vi "VP_NanoPositioner_FPGA_MultiScan.vi"() -> ()   [LabVIEW 2015]
uses:
  FPGA states.ctl
  FPGA Commands.ctl
  RT VIs/Scan type.ctl
  <vilib>/Platform/TimedLoop/XDataNode/timing_clust.ctl
  <vilib>/Platform/TimedLoop/XDataNode/nitl_modes.ctl
  <vilib>/Platform/TimedLoop/XDataNode/wakeup.ctl
  Control X Up Down Ramp.ctl
  Detector_Trigger_Control.ctl
  Control Y Up Down Ramp.ctl
  <vilib>/rvi/Emulation/niFpgaGetClockAttributes.vi
  <vilib>/rvi/Emulation/niFpgaSctlEmulationGetInTimedLoop.vi
  <vilib>/rvi/Emulation/niFpgaEmulationReportErrorSimple.vi
  <vilib>/rvi/Emulation/niFpgaProcessEmulError.vi
  <vilib>/rvi/Emulation/niFpgaCriticalErrorInLSC.vi
  <vilib>/rvi/interface/RandomDataEmulation/niFpgaRandomDataHandleErrors.vi
  <vilib>/rvi/eio/common/nirviEmuTemplateMethod_errors.vi
  <vilib>/rvi/DataTransferAndStorage/Container/XNode/niFpgaContainer.xnode
  <vilib>/rvi/interface/RandomDataEmulation/nirviRandomDataFpgaReadWriteTemplate.vi
  <vilib>/eio/EIONode/EIONode.xnode
  <vilib>/rvi/Analysis/measure/butterworth/XNode/niFpgaButterworthFilter.xnode
  <vilib>/Platform/TimedLoop/XDataNode/XDataNode.xnode
  <vilib>/Platform/TimedLoop/XDataNode/XDNodeRunTimeDep.lvlib
panel:
  in  "Scan type":T1
  out "Interferometer Loop Error":errorcluster
  out "Fly scan completed":bool
  out "Y scan done":bool=TRUE
  out "X scan done":bool=TRUE
  out "Wait error":errorcluster
  out "Shutdown error":errorcluster
  out "FPGA error monitor":errorcluster
  out "Run Loop error":errorcluster
  in  "Wait timer (ms)":u16=50 caption="Count(mSec)"
  in  "New FPGA command":bool
  in  "FPGA command":T2
  out "FPGA state":T3
  out "End Run Error":errorcluster
  out "Measured Data Trigger Time Period (Ticks)":u32
  in  "Data Trigger Time Period (uSec)":u32 caption="Detector Trigger Time Period (uSec)"
  out "Trigger for Data":fxp<+/-,58,25>
  out "Fly Scan Running":bool
  in  "Fly Scan":bool
  out "If True End Y Down Ramp":bool
  in  "Y Ramp Drop Size (nm)":fxp<+/-,16,16>
  out "Ramp Mid Range":bool
  out "If True End Up Ramp":bool
  out "Start or middle":bool=TRUE
  in  "Y Start Marker (nm)":fxp<+/-,58,25> format="%#_55g"
  out "Y Ramp Slope":fxp<+,48,16>
  in  "Y Ramp End (nm)":fxp<+/-,16,16>
  in  "Y Ramp Start (nm)":fxp<+/-,16,16>
  in  "Y Ramp Period (usec)":fxp<+,32,32>
  in  "X Ramp Period (usec)":fxp<+,32,32>
  in  "X Ramp End (nm)":fxp<+/-,16,16>
  in  "X Ramp Start (nm)":fxp<+/-,16,16>
  out "If True End X Down Ramp":bool
  out "X Ramp Mid Range":bool
  out "If True End X Up Ramp":bool
  out "Y Ramp Drop":bool
  out "Next Do Down Ramp":bool
  out "Continue Run":bool
  in  "X Start Marker (nm)":fxp<+/-,58,25>
  out "X Ramp Slope":fxp<+,48,16> format="%.37g"
  in  "DT Reset":bool
  in  "DT Duty Cycle (periods)":fxp<+,32,0>=0.5 caption="DT duty cycle (periods)"
  in  "DT Reference DC Offset (V)":fxp<+/-,16,16>
  in  "DT Reference Amplitude (V)":fxp<+/-,40,17>
  in  "DT Phase Offset (periods)":fxp<+,32,0>
  in  "DT Frequency (periods/tick)":fxp<+,32,0>=0.0002500000409781933
  in  "Trigger Wave Generator":T4(ring)
  out "If True End Trigger Low":bool
  in  "Trigger Low Level (V)":fxp<+/-,20,5>=-5.0
  in  "Trigger High Level (V)":fxp<+/-,20,5>=5.0
  out "If True End Trigger High":bool
  out "Trigger Mid High":bool
  in  "Trigger Low Period (usec)":fxp<+/-,64,45>
  in  "Trigger High Period (usec)":fxp<+/-,64,45>
  out "Measured Z Reference Time Period (Ticks)":u32
  in  "Z Reference Time Period (uSec)":u32
  in  "Z White Noise Amplitude":u16=32767
  in  "Z White Noise Seed":u32=4
  in  "Z Phase Offset (periods)":fxp<+,32,0>
  in  "Z Frequency (periods/tick)":fxp<+,32,0>=0.0002500000409781933
  in  "Z Reference DC Offset (nm)":fxp<+/-,16,16>
  in  "Z Reference Amplitude (nm)":fxp<+/-,40,17>
  in  "Z Reference Reset":bool
  in  "Z Reference Wave Selection":T5(ring)
  in  "Y White Noise Amplitude":u16=32767
  in  "Y White Noise Seed":u32=4
  out "Measured Y Reference Time Period (Ticks)":u32
  in  "Y Reference Time Period (uSec)":u32
  in  "Y Reference Reset":bool
  in  "Y Reference Wave Selection":T6(ring)
  in  "Detector Trigger Lower Limit (V)":fxp<+/-,20,5>=-5.0
  out "Detector Trigger In Range?":bool
  in  "Detector Trigger Upper Limit (V)":fxp<+/-,20,5>=5.0
  out "Detector Trigger (V)":fxp<+/-,20,5> format="%.29g"
  out "Measured Detector Trigger Time Period (Ticks)":u32
  in  "Detector Trigger Time Period (uSec)":u32
  out "Measured Trigger Gen Time Period (Ticks)":u32
  in  "Trigger Generation Time Period (uSec)":u32
  in  "Reference Signal Source":T7(ring)
  in  "Z-Stage Scaling Direction":fxp<+/-,3,3>=-1.0
  in  "Y-Stage Scaling Direction":fxp<+/-,3,3>=-1.0
  in  "Y Phase Offset (periods)":fxp<+,32,0>
  in  "Y Frequency (periods/tick)":fxp<+,32,0>=0.0002500000409781933
  in  "Optics and or Sample Stage":T8(ring)
  out "Z Stage External Reference (nm)":fxp<+/-,58,25>
  in  "Mod 3 AI2 V to nm Scaling":fxp<+,47,18>
  out "Mod 8 Input AI2 (V)":fxp<+/-,24,5>
  out "Y Stage External Reference (nm)":fxp<+/-,58,25>
  in  "Mod 3 AI1 V to nm Scaling":fxp<+,47,18>
  out "Mod 8 Input AI1 (V)":fxp<+/-,24,5>
  in  "Sample Z Stage Resolution (nm)":fxp<+,33,3>=0.001000046730041504
  in  "Sample Y Stage Resolution (nm)":fxp<+,33,3>=0.001000046730041504
  in  "Sample X Stage Resolution (nm)":fxp<+,33,3>=0.001000046730041504
  out "Sample Z Stage Displacement (nm)":fxp<+/-,58,25>
  out "Sample Z Stage Displacement raw (nm)":fxp<+/-,64,35> format="%.62g"
  out "Sample Y Stage Displacement (nm)":fxp<+/-,58,25>
  out "Sample Y Stage Displacement raw (nm)":fxp<+/-,64,35> format="%.41g"
  out "Sample X Stage Displacement raw (nm)":fxp<+/-,64,35> format="%.62g"
  out "Sample X Stage Displacement (nm)":fxp<+/-,58,25>
  in  "Reset Sample Z":bool
  out "32 bit Count Sample  Z":i32
  in  "Reset Sample Y":bool
  out "32 bit Count Sample  Y":i32
  in  "Reset Sample X":bool
  out "32 bit Count Sample X":i32
  out "Mod6/DIO3":bool
  out "Mod6/DIO2":bool
  out "Mod5/DIO3":bool
  out "Mod5/DIO2":bool
  out "Mod4/DIO3":bool
  out "Mod4/DIO2":bool
  out "Measured Analog Input Time Period (Ticks)":u32
  in  "Analog Input Time Period (uSec)":u32
  out "X Stage External Reference (nm)":fxp<+/-,58,25>
  in  "Mod 3 AI0 V to nm Scaling":fxp<+,47,18>
  out "Mod 3 Input AI0 (V)":fxp<+/-,24,5>
  in  "X-Stage Scaling Direction":fxp<+/-,3,3>=-1.0
  in  "Z-Stage nm to V Scaling":fxp<+/-,32,12>
  in  "Y-Stage nm to V Scaling":fxp<+/-,32,12>
  in  "X-Stage nm to V Scaling":fxp<+/-,32,12>
  out "Kxx Output, Kxx*ex (V)":fxp<+/-,58,25>
  out "Kyy Output, Kyy*ey (V)":fxp<+/-,58,25>
  out "Kzz Output, Kzz*ez (V)":fxp<+/-,58,25>
  in  "sos gain SF Controller xx1":fxp<+/-,42,9>
  in  "-a01(2) xx1":fxp<+/-,64,9>[](array[numeric])=[0.0, 0.0, 0.0, 0.0, 0.0, 0.0, 0.0, 0.0, 0.0, 0.0, 0.0, 0.0, 0.0, 0.0, 0.0, 0.0, 0.0, 0.0, 0.0, 0.0]
  in  "-a02(2) xx1":fxp<+/-,64,9>[](array[numeric])=[0.0, 0.0, 0.0, 0.0, 0.0, 0.0, 0.0, 0.0, 0.0, 0.0, 0.0, 0.0, 0.0, 0.0, 0.0, 0.0, 0.0, 0.0, 0.0, 0.0]
  in  "b01(2) xx1":fxp<+/-,64,9>[](array[numeric])=[0.0, 0.0, 0.0, 0.0, 0.0, 0.0, 0.0, 0.0, 0.0, 0.0, 0.0, 0.0, 0.0, 0.0, 0.0, 0.0, 0.0, 0.0, 0.0, 0.0]
  in  "b02(2) xx1":fxp<+/-,64,9>[](array[numeric])=[0.0, 0.0, 0.0, 0.0, 0.0, 0.0, 0.0, 0.0, 0.0, 0.0, 0.0, 0.0, 0.0, 0.0, 0.0, 0.0, 0.0, 0.0, 0.0, 0.0]
  in  "sos gain SF Controller yy1":fxp<+/-,42,9>
  in  "-a01(2) yy1":fxp<+/-,64,9>[](array[numeric])=[0.0, 0.0, 0.0, 0.0, 0.0, 0.0, 0.0, 0.0, 0.0, 0.0, 0.0, 0.0, 0.0, 0.0, 0.0, 0.0, 0.0, 0.0, 0.0, 0.0]
  in  "-a02(2) yy1":fxp<+/-,64,9>[](array[numeric])=[0.0, 0.0, 0.0, 0.0, 0.0, 0.0, 0.0, 0.0, 0.0, 0.0, 0.0, 0.0, 0.0, 0.0, 0.0, 0.0, 0.0, 0.0, 0.0, 0.0]
  in  "b01(2) yy1":fxp<+/-,64,9>[](array[numeric])=[0.0, 0.0, 0.0, 0.0, 0.0, 0.0, 0.0, 0.0, 0.0, 0.0, 0.0, 0.0, 0.0, 0.0, 0.0, 0.0, 0.0, 0.0, 0.0, 0.0]
  in  "b02(2) yy1":fxp<+/-,64,9>[](array[numeric])=[0.0, 0.0, 0.0, 0.0, 0.0, 0.0, 0.0, 0.0, 0.0, 0.0, 0.0, 0.0, 0.0, 0.0, 0.0, 0.0, 0.0, 0.0, 0.0, 0.0]
  in  "sos gain SF Controller zz1":fxp<+/-,42,9>
  in  "-a01(2) zz1":fxp<+/-,64,9>[](array[numeric])=[0.0, 0.0, 0.0, 0.0, 0.0, 0.0, 0.0, 0.0, 0.0, 0.0, 0.0, 0.0, 0.0, 0.0, 0.0, 0.0, 0.0, 0.0, 0.0, 0.0]
  in  "-a02(2) zz1":fxp<+/-,64,9>[](array[numeric])=[0.0, 0.0, 0.0, 0.0, 0.0, 0.0, 0.0, 0.0, 0.0, 0.0, 0.0, 0.0, 0.0, 0.0, 0.0, 0.0, 0.0, 0.0, 0.0, 0.0]
  in  "b01(2) zz1":fxp<+/-,64,9>[](array[numeric])=[0.0, 0.0, 0.0, 0.0, 0.0, 0.0, 0.0, 0.0, 0.0, 0.0, 0.0, 0.0, 0.0, 0.0, 0.0, 0.0, 0.0, 0.0, 0.0, 0.0]
  in  "b02(2) zz1":fxp<+/-,64,9>[](array[numeric])=[0.0, 0.0, 0.0, 0.0, 0.0, 0.0, 0.0, 0.0, 0.0, 0.0, 0.0, 0.0, 0.0, 0.0, 0.0, 0.0, 0.0, 0.0, 0.0, 0.0]
  in  "Scaling mV to V":fxp<+,33,10>=0.0009765625
  in  "System Loop Type":enum16{"Open Loop", "Closed Loop"}(ring)
  in  "Timeout FPGA FIFO1":i32=40000000
  out "FIFO Timed Out":bool
  out "Number of Data Strings":i32
  in  "Y Reference DC Offset (nm)":fxp<+/-,16,16>
  in  "X Reference DC Offset (nm)":fxp<+/-,16,16>
  in  "Y Reference Amplitude (nm)":fxp<+/-,40,17>
  out "Z Stage Reference (nm)":fxp<+/-,58,25> format="%.41g"
  out "Y Stage Reference (nm)":fxp<+/-,58,25> format="%.41g"
  out "Optics Z Stage Displacement (nm)":fxp<+/-,58,25>
  out "Optics Z Stage Displacement raw (nm)":fxp<+/-,64,35>
  in  "Optics Z Stage Resolution (nm)":fxp<+,33,3>=0.001000046730041504
  in  "Reset Optics Z":bool
  out "32 bit Count Optics  Z":i32
  out "Mod6/DIO1":bool
  out "Mod6/DIO0":bool
  out "Optics Y Stage Displacement (nm)":fxp<+/-,58,25>
  out "Optics Y Stage Displacement raw (nm)":fxp<+/-,64,35>
  in  "Optics Y Stage Resolution (nm)":fxp<+,33,3>=0.001000046730041504
  in  "Reset Optics Y":bool
  out "32 bit Count Optics  Y":i32
  out "Mod5/DIO1":bool
  out "Mod5/DIO0":bool
  out "Z-Stage Input In Range?":bool
  out "Y-Stage Input In Range?":bool
  in  "Controller Output Lower Limit":fxp<+/-,20,5>=-5.0
  out "X-Stage Input In Range?":bool
  in  "Controller Output Upper Limit":fxp<+/-,20,5>=5.0
  in  "X White Noise Amplitude":u16=32767
  in  "X White Noise Seed":u32=4
  in  "X Reference Reset":bool
  in  "X Reference Wave Selection":T9(ring)
  out "Measured Counter Time Period (Ticks)":u32
  out "Measured Datalog Time Period (Ticks)":u32
  out "Measured Plant Output Time Period (Ticks)":u32
  out "Measured Controller Output Time Period (Ticks)":u32
  out "Measured Controller Time Period (Ticks)":u32
  out "Measured X Reference Time Period (Ticks)":u32
  out "Optics X Stage Displacement raw (nm)":fxp<+/-,64,35>
  in  "Optics X Stage Resolution (nm)":fxp<+,33,3>=0.001000046730041504 format="%#_31g"
  in  "Plant Output Time Period (uSec)":u32
  out "Optics X Stage Displacement (nm)":fxp<+/-,58,25>
  in  "Reset Optics X":bool
  out "32 bit Count Optics X":i32
  out "Mod4/DIO1":bool
  out "Mod4/DIO0":bool
  out "Start Run Error":errorcluster
  out "stop case":bool
  in  "Controller Output Time Period (uSec)":u32
  in  "Datalog Cases":T10(ring)
  out "PI Z-Stage Input (V)":fxp<+/-,20,5> format="%.29g"
  out "PI Y-Stage Input (V)":fxp<+/-,20,5> format="%.29g"
  out "PI X-Stage Input (V)":fxp<+/-,20,5> format="%.29g"
  in  "Controller Time Period (uSec)":u32
  in  "Datalog Time Period (uSec)":u32
  in  "X Reference Time Period (uSec)":u32
  in  "X Reference Amplitude (nm)":fxp<+/-,40,17>
  out "X Stage Reference (nm)":fxp<+/-,58,25> format="%.41g"
  out "FIFO Timed Out?":bool
  in  "X Phase Offset (periods)":fxp<+,32,0>
  in  "X Frequency (periods/tick)":fxp<+,32,0>=0.0002500000409781933
types:
  T1 = typedef "Scan type.ctl" = enum16{"Fly", "Step"}
  T2 = typedef "FPGA Commands.ctl" = enum16{"Start Scan", "Shutdown"}
  T3 = typedef "FPGA states.ctl" = enum16{"Wait", "Start Run", "Run", "End Run", "Shutdown"}
  T4 = enum16{"Custom Square Wave ", "Square Wave 1", "Square Wave 2"}
  T5 = enum16{"Constant", "Sine Wave", "Sawtooth Wave", "Square Wave", "Filtered White Noise"}
  T6 = enum16{"Constant", "Sine Wave", "Custom Ramp Wave", "Filtered White Noise"}
  T7 = enum16{"FPGA Generated Reference", "External Reference"}
  T8 = enum16{"Optics Stage Only", "Optics and Sample Stage"}
  T9 = enum16{"Constant", "Sine Wave", "Custom Up Down Ramp", "Filtered White Noise"}
  T10 = enum16{"Data Log 1", "Data Log 2", "Data Log 3", "Data Log 4", "Data Log 5", "Data Log 6", "Data Log 7", "Data Log 8", "Data Log 9", "Data Log 10", "Data Log 11", "Data Log 12", "Data Log 13", "Data Log 14", "Data Log 15", "Data Log 16"}
  T11 = typedef "Control Y Up Down Ramp.ctl" = enum16{"Y Up Ramp", "Y Down Ramp"}
  T12 = typedef "Detector_Trigger_Control.ctl" = enum16{"Trigger High", "Trigger Low"}
  T13 = typedef "Control X Up Down Ramp.ctl" = enum16{"X Up Ramp", "X Down Ramp"}
  T14 = typedef "XDNodeRunTimeDep.lvlib/timing_clust.ctl" = cluster{"Expected End [f-1]":u64, "Actual End [f-1]":u64, "Finished Late? [f-1]":bool, "Expected End [i-1]":u64, "Actual End [i-1]":u64, "Finished Late? [i-1]":bool, "Expected Start [i]":u64, "Actual Start [i]":u64, "Expected Start [f]":u64, "Actual Start [f]":u64, "Source Name":string, "Structure Name":string, "Period":i64, "Deadline":i64, "Offset":i64, "Start":i64, "Priority":i32, "Timeout":i32, "Mode":T15, "Wakeup Reason":T16, "Error":errorcluster, "Source Type":string, "Secondary Source Type":string, "Global End Time":u64, "Global Start Time":u64, "Frame Duration":u64, "Iteration Duration":u64, "Assigned CPU":i32, "I/O Scan Engine Mode":u32}
  T15 = typedef "XDNodeRunTimeDep.lvlib/nitl_modes.ctl" = enum32{"No Change", "Process missed periods, maintain original phase", "Discard missed periods, maintain original phase", "Process missed periods, ignore original phase", "Discard missed periods, ignore original phase"}
  T16 = typedef "XDNodeRunTimeDep.lvlib/wakeup.ctl" = enum32{"Normal", "Aborted", "Asynchronous wakeup", "Timing source error", "Timed loop error", "Timeout"}
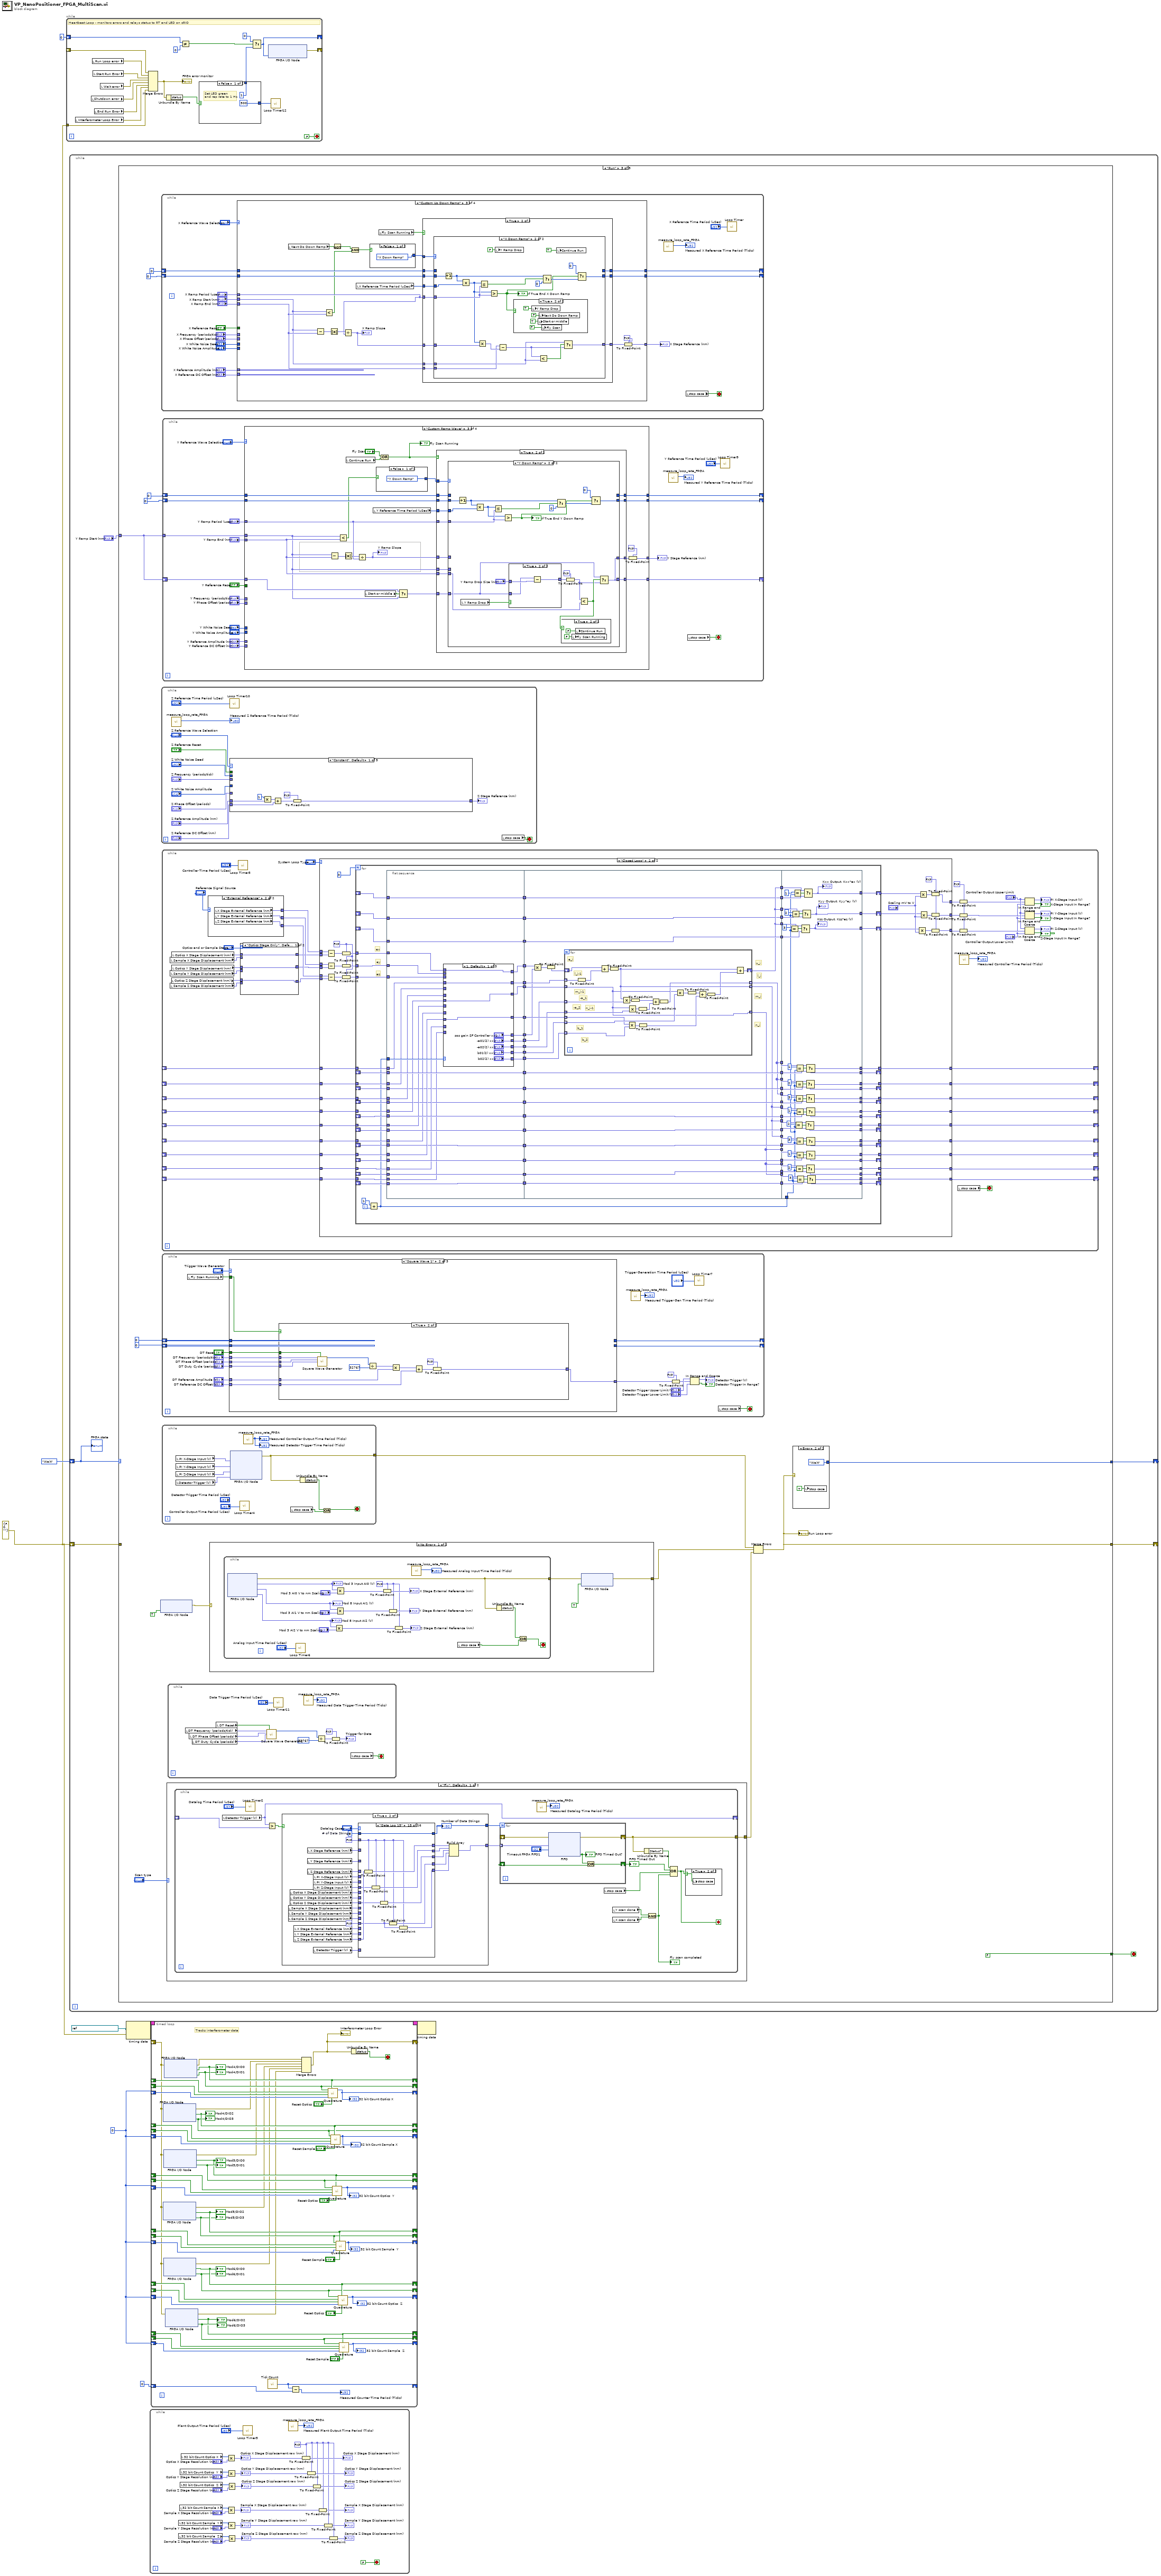
[diagram p0: block diagram]
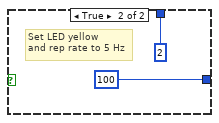
[diagram p2: hidden frame]
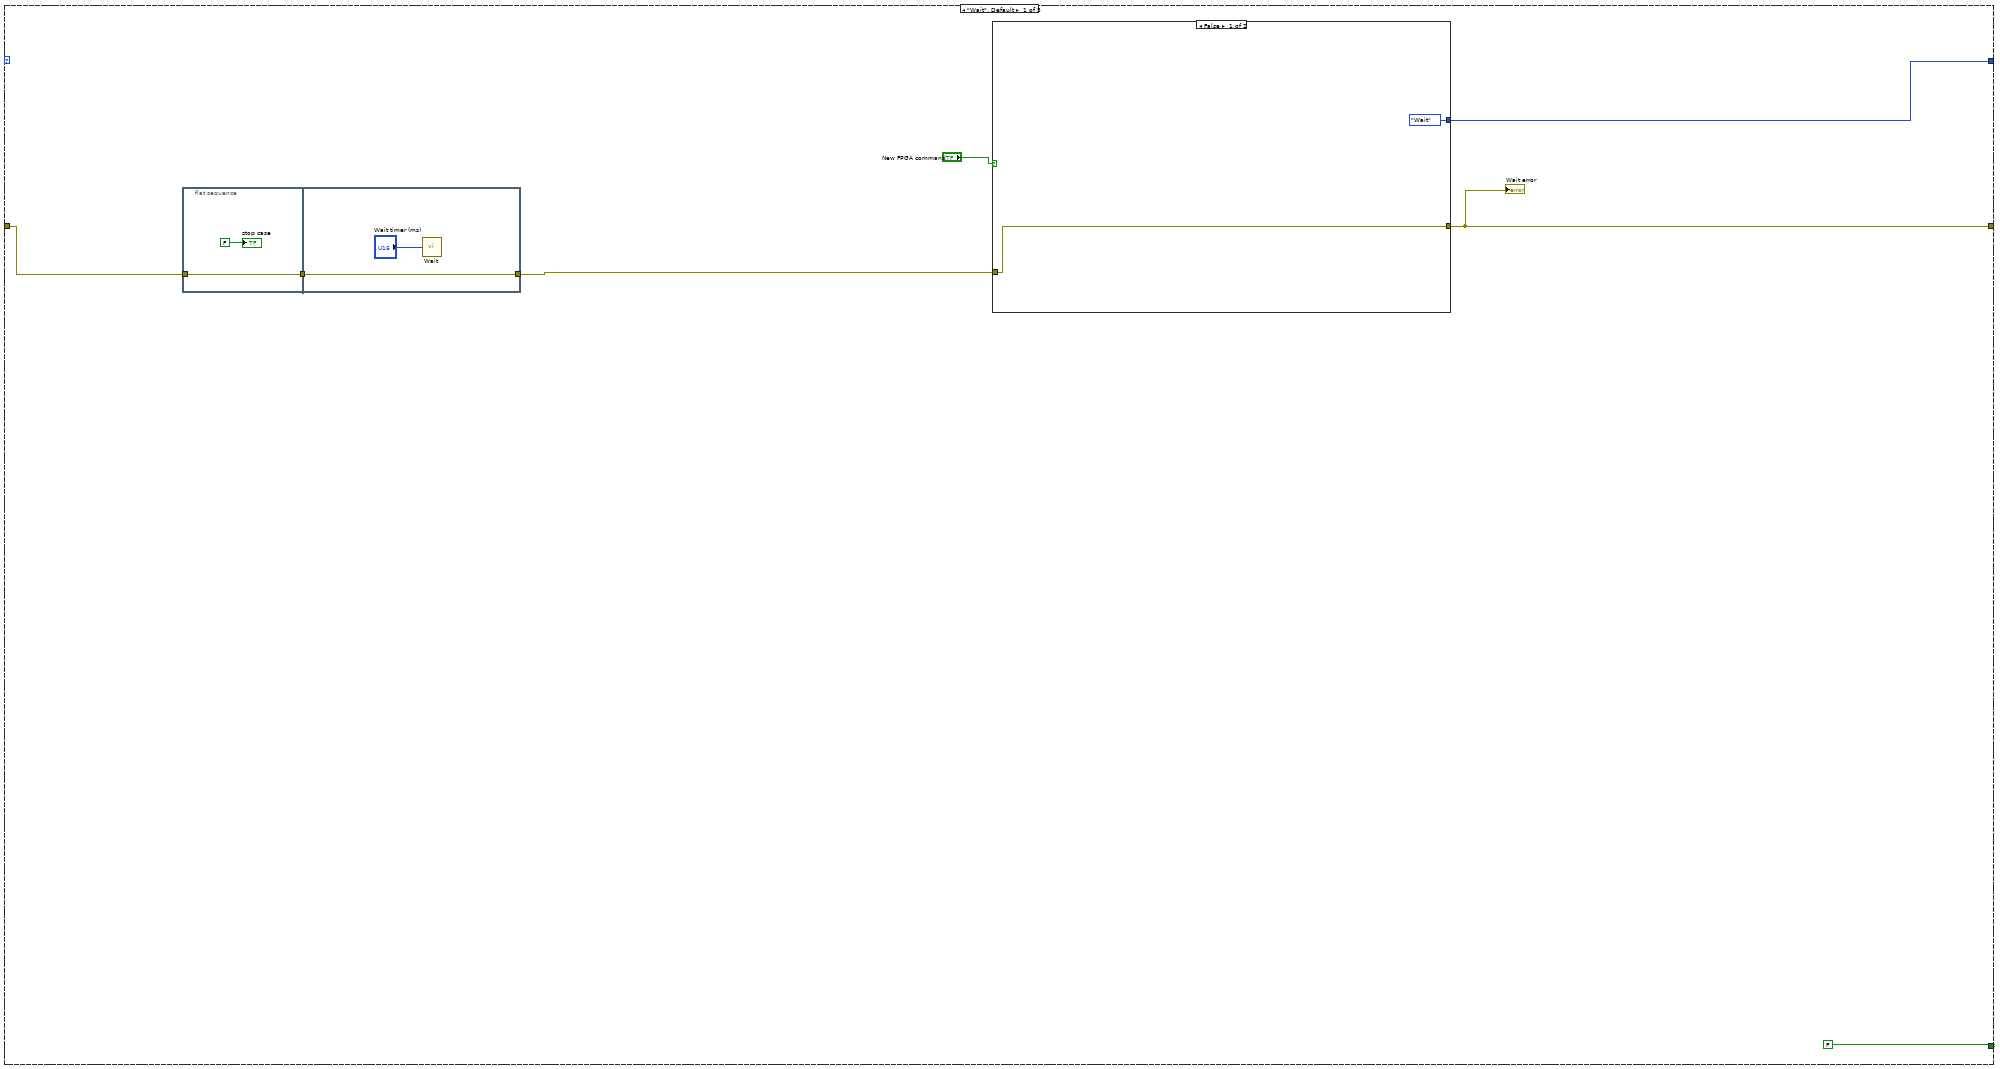
[diagram p3: hidden frame]
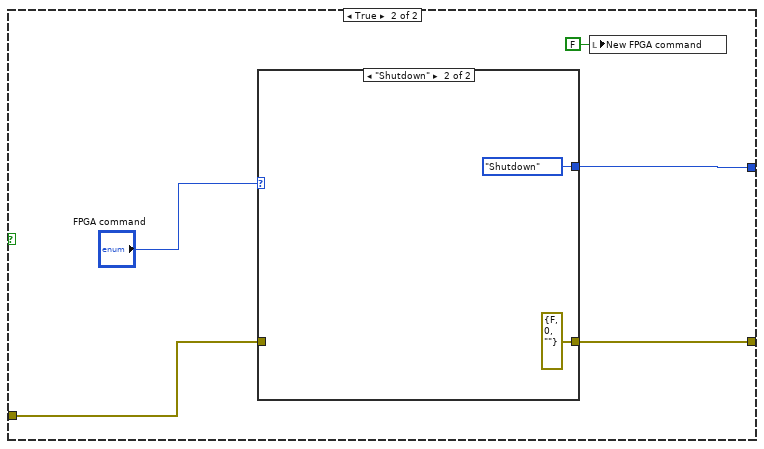
[diagram p4: hidden frame]
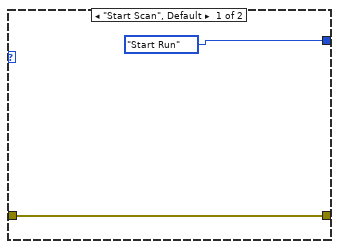
[diagram p5: hidden frame]
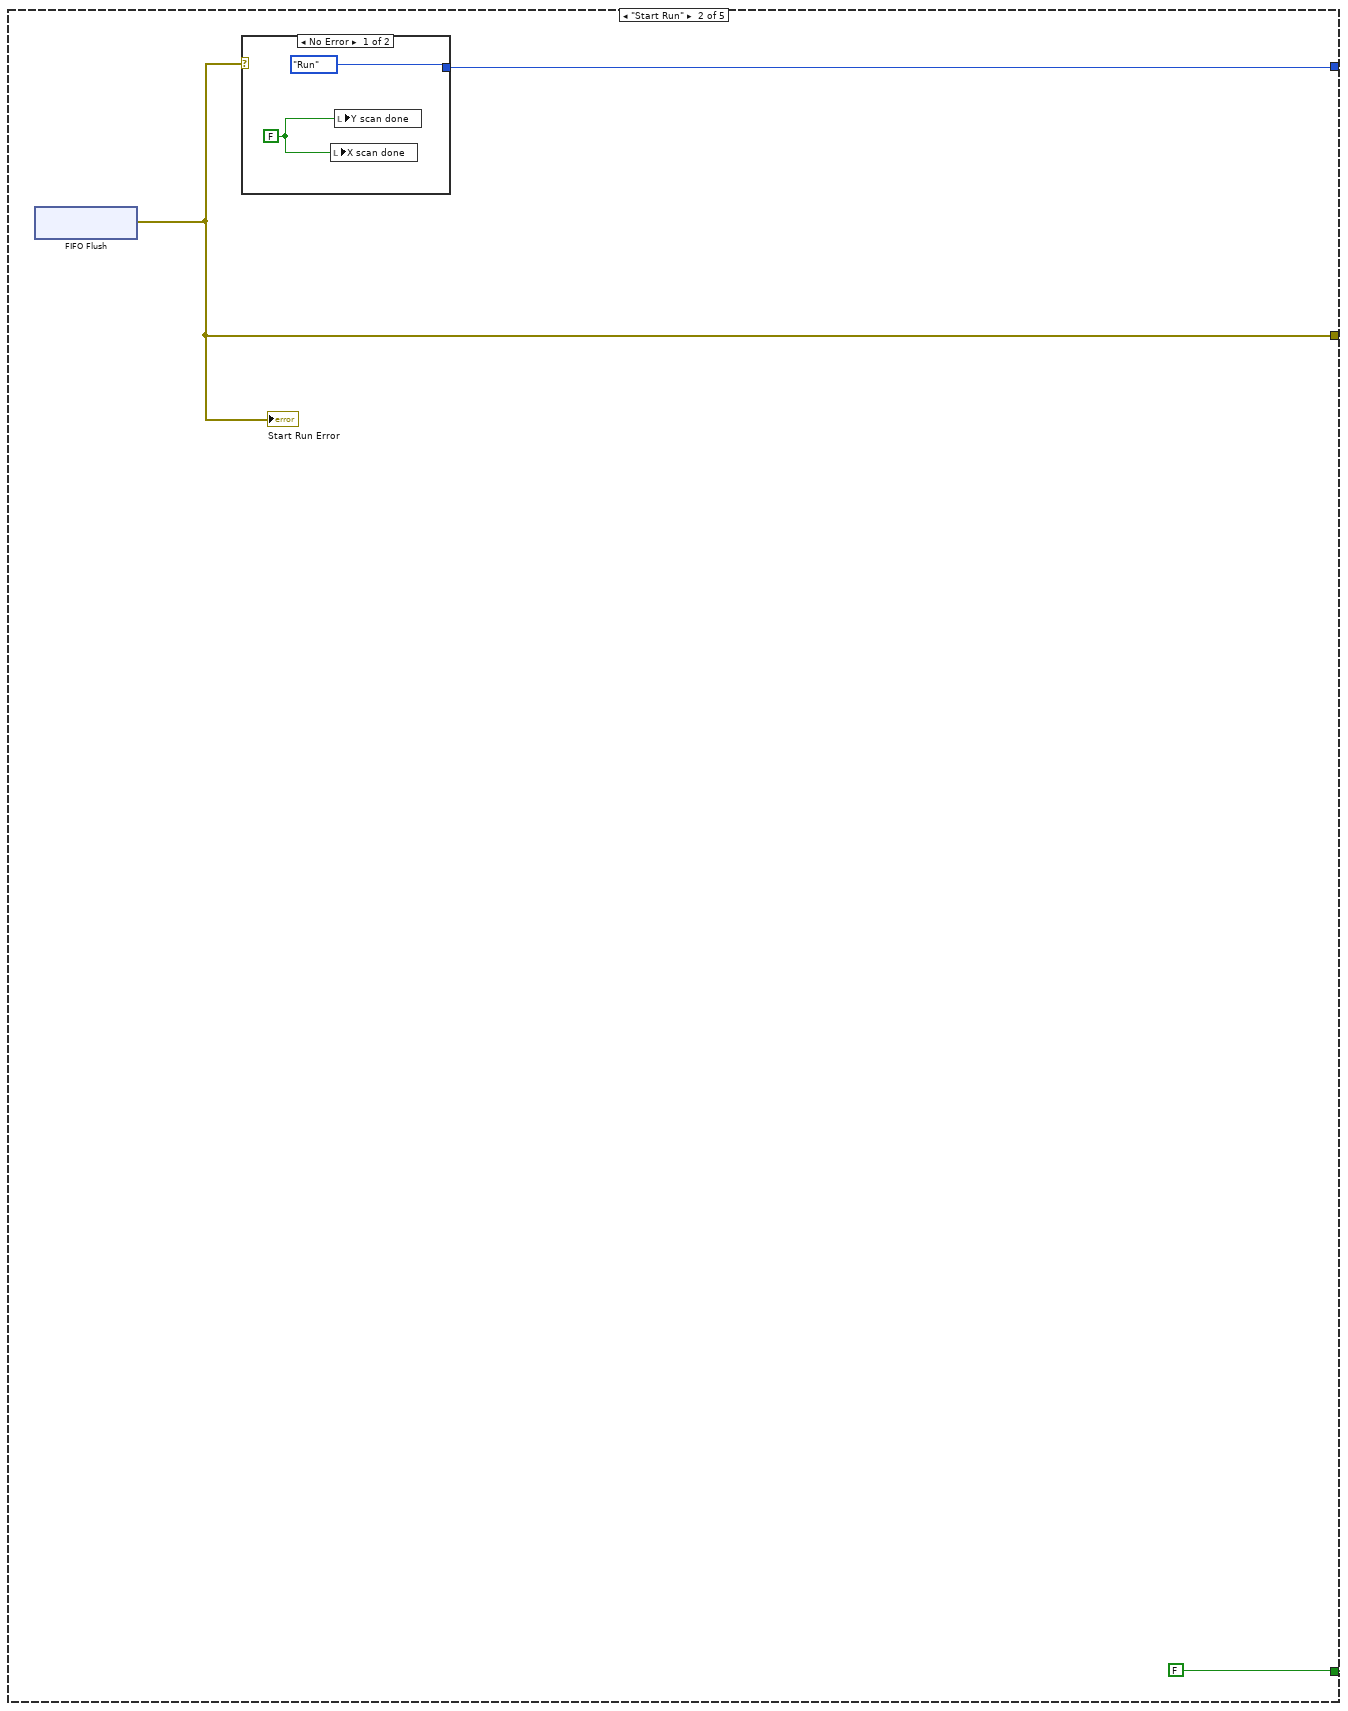
[diagram p6: hidden frame]
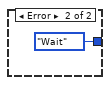
[diagram p7: hidden frame]
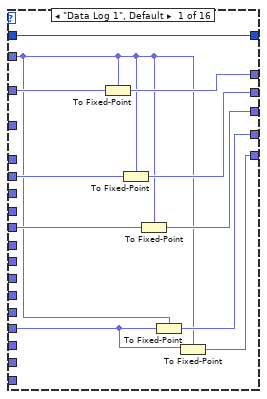
[diagram p10: hidden frame]
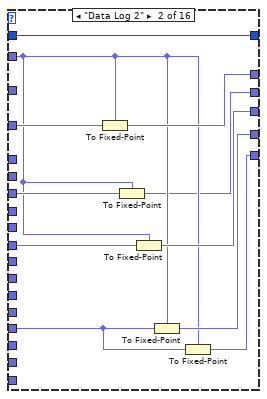
[diagram p11: hidden frame]
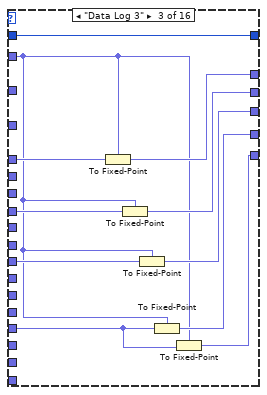
[diagram p12: hidden frame]
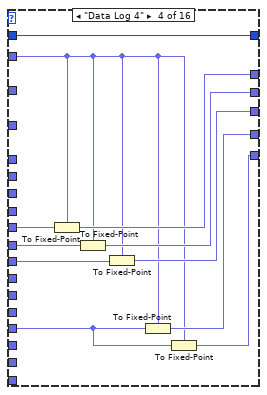
[diagram p13: hidden frame]
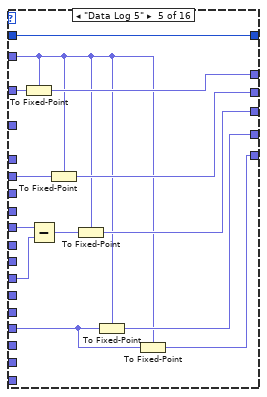
[diagram p14: hidden frame]
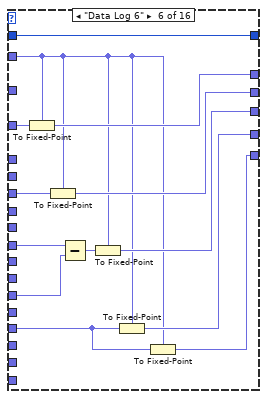
[diagram p15: hidden frame]
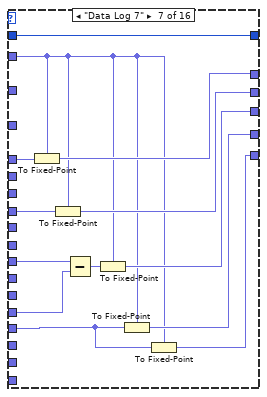
[diagram p16: hidden frame]
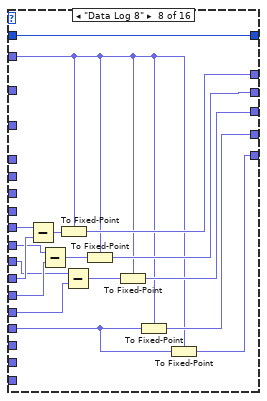
[diagram p17: hidden frame]
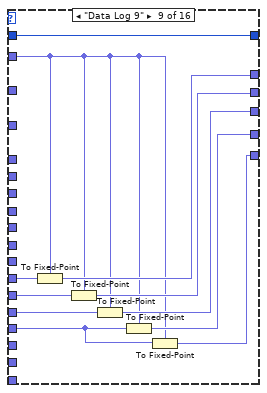
[diagram p18: hidden frame]
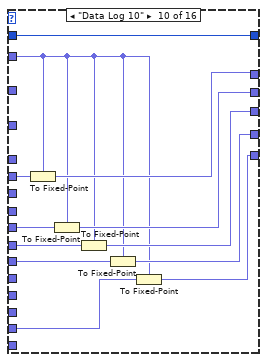
[diagram p19: hidden frame]
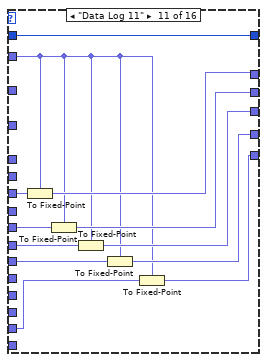
[diagram p20: hidden frame]
diagram:
  w4 = 0 ("Tick Count(Ticks)")
  w1 = errorcluster {"status"=FALSE, "code"=0, "source"=""} ("error IO")
  n1 = while {
    tunnel: w1 -> [w22]
    shift-right: [w20] -> _
    shift-left: _ -> [w19]
    shift-right: [w17] -> _
    shift-left: u8 0 ("USER FPGA LED") -> [w15]
    stop <- FALSE stop-if-true
    # "Heartbeat Loop - monitors errors and relays status to RT and LED on cRIO"
    n2 = local read "Interferometer Loop Error"() -> (w9:errorcluster)
    n3 = local read "Shutdown error"() -> (w24:errorcluster)
    n4 = local read "Run Loop error"() -> (w27:errorcluster)
    n5 = local read "Start Run Error"() -> (w26:errorcluster)
    n6 = local read "End Run Error"() -> (w23:errorcluster)
    n7 = local read "Wait error"() -> (w25:errorcluster)
    n8 = Merge Errors(w19, w27, w26, w25, w24, w23, w9, w22) -> (w21:errorcluster)
    "FPGA error monitor" <- w21
    n9 = Unbundle By Name(w21) -> ("status"=w10:bool)
    n10 = Not Equal?(x=w15, y=u8 0) -> (x != y?=w13:bool)
    n11 = case shown="False" w10 {
      tunnel: [u16 500 ("Count(mSec)") u16 100 ("Count(mSec)")] -> w18
      tunnel: [u8 1 ("USER FPGA LED") u8 2 ("USER FPGA LED")] -> w11
      frame False {
        # "Set LED green \nand rep rate to 1 Hz"
      }
      frame True {
        # "Set LED yellow \nand rep rate to 5 Hz"
      }
    }
    n12 = Select(t=u8 0, s=w13, f=w11) -> (s? t:f=w17:u8)
    n13 = xnode "FPGA I/O Node"("USER FPGA LED"=w17) -> ("error out"=w20:errorcluster)  [unwired: 2 in, 1 out]
    n14 = call "Loop Timer12"("Count(mSec)"=w18) -> ()  [unwired: 1 out]
  }
  n15 = while {
    shift-right: [w35] -> _
    shift-left: FPGA_states."Wait" -> [w37]
    shift-right: [w32] -> _
    shift-left: w1 -> [w34]
    stop <- w36 stop-if-true
    n16 = case shown="\"Run\"" w37 {
      tunnel: [w43 w60 w71 w1303 w1307] -> w32
      tunnel: [FALSE FALSE FALSE FALSE TRUE] -> w36
      tunnel: [w38 w61 w72 FPGA_states."Wait" FPGA_states."Shutdown"] -> w35
      tunnel: w34 -> [w40 _ _ w1303 w1308]
      tunnel: "Y Ramp Start (nm)" -> [_ _ w69 _ _]
      frame "Wait", Default {
        n17 = flat-sequence {
          tunnel: w40 -> [w45]
          tunnel: [w45] -> w41
          tunnel: [w47] -> w39
          tunnel: w41 -> [w47]
          frame #0 {
            "stop case" <- FALSE ("stop case")
          }
          frame #1 {
            n18 = call "Wait"("Count(mSec)"="Wait timer (ms)") -> ()  [unwired: 1 out]
          }
        }
        n19 = case shown="False" "New FPGA command" {
          tunnel: [FPGA_states."Wait" w55] -> w38
          tunnel: w39 -> [w50 w54]
          tunnel: [w50 w53] -> w43
          frame False {
          }
          frame True {
            n20 = case shown="\"Shutdown\"" "FPGA command" {
              tunnel: [FPGA_states."Start Run" FPGA_states."Shutdown"] -> w55
              tunnel: w54 -> [w56 _]
              tunnel: [w56 errorcluster {"status"=FALSE, "code"=0, "source"=""} ("error IO")] -> w53
              frame "Start Scan", Default {
              }
              frame "Shutdown" {
              }
            }
            n21 = local write "New FPGA command"(FALSE ("New FPGA command")) -> ()
          }
        }
        "Wait error" <- w43
      }
      frame "Start Run" {
        n22 = xnode ("FIFO Flush")() -> ("error out"=w60:errorcluster)  [unwired: 2 in, 1 out]
        "Start Run Error" <- w60
        n23 = case shown="No Error" w60 {
          tunnel: [FPGA_states."Run" FPGA_states."Wait"] -> w61
          frame No Error {
            w63 = FALSE
            n24 = local write "X scan done"(w63) -> ()
            n25 = local write "Y scan done"(w63) -> ()
          }
          frame Error {
          }
        }
      }
      frame "Run" {
        n26 = xnode "FPGA I/O Node"("Mod3/Start"=TRUE ("I/O Item")) -> ("error out"=w67:errorcluster)  [unwired: 2 in, 1 out]
        n27 = while {
          shift-right: [w1165] -> _
          shift-left: u32 0 ("f") -> [w1163]
          shift-right: [w1164] -> _
          shift-left: u32 0 -> [w1162]
          stop <- w1174 stop-if-true
          n28 = case shown="\"Custom Up Down Ramp\"" "X Reference Wave Selection" {
            tunnel: "X Frequency (periods/tick)" -> [_ w1196 _ _]
            tunnel: "X Phase Offset (periods)" -> [_ w1195 _ _]
            tunnel: "X Reference Reset" -> [_ w1193 _ w1292]
            tunnel: "X White Noise Seed" -> [_ _ _ w1294]
            tunnel: "X White Noise Amplitude" -> [_ _ _ w1291]
            tunnel: "X Reference Amplitude (nm)" -> [w1181 w1188 _ w1282]
            tunnel: "X Reference DC Offset (nm)" -> [w1180 w1187 _ w1283]
            tunnel: [w1179 w1186 w1200 w1285] -> w1167
            tunnel: [_ _ w1213 _] -> w1165
            tunnel: [_ _ w1212 _] -> w1164
            tunnel: w1163 -> [_ _ w1211 _]
            tunnel: w1162 -> [_ _ w1210 _]
            tunnel: "X Ramp Period (usec)" -> [_ _ w1209 _]
            tunnel: "X Ramp Start (nm)" -> [_ _ w1198 _]
            tunnel: "X Ramp End (nm)" -> [_ _ w1199 _]
            frame "Constant", Default {
              n29 = Multiply(x=i16 1 ("y"), y=w1181) -> (x*y=w1184:fxp<+/-,56,33>)
              n30 = Add(x=w1184, y=w1180) -> (x+y=w1183:fxp<+/-,56,33>)
              n31 = To Fixed-Point(fixed-point type=fxp<+/-,58,25> 0.0, number=w1183) -> (fixed-point=w1179:fxp<+/-,58,25>)
            }
            frame "Sine Wave" {
              n32 = call "Sine Wave Generator"("frequency (periods/tick)"=w1196, "reset"=w1193, "phase offset (periods)"=w1195) -> ("sine out"=w1194:i16)  [unwired: 12 in]
              n33 = Divide(x=w1194, y=i16 32767) -> (x/y=w1189:fxp<+/-,41,18>)
              n34 = Multiply(x=w1189, y=w1188) -> (x*y=w1191:fxp<+/-,64,35>)
              n35 = Add(x=w1191, y=w1187) -> (x+y=w1190:fxp<+/-,64,36>)
              n36 = To Fixed-Point(fixed-point type=fxp<+/-,58,25> 0.0, number=w1190) -> (fixed-point=w1186:fxp<+/-,58,25>)
            }
            frame "Custom Up Down Ramp" {
              n37 = local read "Next Do Down Ramp"() -> (w1205:bool)
              n38 = Subtract(x=w1198, y=w1199) -> (x-y=w1215:fxp<+/-,17,17>)
              n39 = Less?(x=w1198, y=w1199) -> (x < y?=w1204:bool)
              n40 = Absolute Value(x=w1215) -> (abs(x)=w1214:fxp<+,16,16>)
              n41 = Not(x=w1205) -> (.not. x?=w1206:bool)
              n42 = Divide(x=w1214, y=w1209) -> (x/y=w1216:fxp<+,48,16>)
              "X Ramp Slope" <- w1216
              n43 = Compound Arithmetic op=AND(w1206, w1204) -> (w1207:bool)
              n44 = local read "X Reference Time Period (uSec)"() -> (w1208:u32)
              n45 = case shown="False" w1207 {
                tunnel: [Control_X_Up_Down_Ramp."X Down Ramp" Control_X_Up_Down_Ramp."X Up Ramp"] -> w1203
                frame False {
                }
                frame True {
                }
              }
              n46 = local read "Fly Scan Running"() -> (w1202:bool)
              n47 = case shown="True" w1202 {
                tunnel: w1203 -> [_ w1233]
                tunnel: w1208 -> [_ w1232]
                tunnel: ["X Start Marker (nm)" w1231] -> w1201
                tunnel: w1209 -> [_ w1230]
                tunnel: w1216 -> [_ w1229]
                tunnel: w1198 -> [_ w1228]
                tunnel: w1199 -> [_ w1227]
                tunnel: [_ w1226] -> w1213
                tunnel: [_ w1225] -> w1212
                tunnel: w1211 -> [_ w1224]
                tunnel: w1210 -> [_ w1223]
                frame False {
                  n48 = local write "Next Do Down Ramp"(FALSE ("Restart Up Ramp")) -> ()
                  n49 = local write "Y Ramp Drop"(FALSE ("Y Toggle 1")) -> ()
                  "X scan done" <- TRUE
                }
                frame True {
                  n50 = case shown="\"X Down Ramp\"" w1233 {
                    tunnel: [w1252 _] -> w1226
                    tunnel: w1224 -> [w1251 _]
                    tunnel: w1232 -> [w1248 w1273]
                    tunnel: w1230 -> [w1247 w1269]
                    tunnel: w1228 -> [w1238 w1260]
                    tunnel: w1227 -> [w1236 w1261]
                    tunnel: [_ w1276] -> w1225
                    tunnel: w1223 -> [_ w1275]
                    tunnel: w1229 -> [w1243 w1267]
                    tunnel: [w1240 w1263] -> w1231
                    frame "X Up Ramp", Default {
                      n51 = Increment(x=w1251) -> (x+1=w1249:u32)
                      n52 = Multiply(x=w1249, y=w1248) -> (x*y=w1244:u32)
                      n53 = Multiply(x=w1244, y=w1243) -> (x*y=w1242:fxp<+,64,48>)
                      n54 = Less Or Equal?(x=w1244, y=w1247) -> (x <= y?=w1246:bool)
                      "X Ramp Mid Range" <- w1246
                      n55 = Add(x=w1242, y=w1238) -> (x+y=w1241:fxp<+/-,64,50>)
                      n56 = Greater?(x=w1244, y=w1247) -> (0:w1237:bool)
                      "If True End X Up Ramp" <- w1237
                      n57 = local write "Y Ramp Drop"(FALSE ("Y Ramp Drop")) -> ()
                      n58 = case shown="True" w1237 {
                        frame False {
                        }
                        frame True {
                          n59 = local write "Start or middle"(TRUE ("Start or middle")) -> ()
                          n60 = local write "Fly Scan"(FALSE ("Fly Scan Start")) -> ()
                          "Y Ramp Drop" <- TRUE ("Boolean")
                          "Next Do Down Ramp" <- TRUE
                        }
                      }
                      n61 = Greater?(x=w1241, y=w1236) -> (0:w1239:bool)
                      n62 = Select(t=w1249, s=w1246, f=u32 0) -> (s? t:f=w1250:u32)
                      n63 = Select(t=w1236, s=w1239, f=w1241) -> (s? t:f=w1240:fxp<+/-,64,50>)
                      n64 = Select(t=u32 0, s=w1237, f=w1250) -> (s? t:f=w1252:u32)
                      "Continue Run" <- TRUE ("Fly Scan Running")
                    }
                    frame "X Down Ramp" {
                      n65 = Increment(x=w1275) -> (x+1=w1274:u32)
                      n66 = Multiply(x=w1274, y=w1273) -> (x*y=w1268:u32)
                      n67 = Multiply(x=w1268, y=w1267) -> (x*y=w1266:fxp<+,64,48>)
                      n68 = Less Or Equal?(x=w1268, y=w1269) -> (x <= y?=w1272:bool)
                      n69 = Greater?(x=w1268, y=w1269) -> (0:w1262:bool)
                      "If True End X Down Ramp" <- w1262
                      n70 = local write "Y Ramp Drop"(FALSE ("Y Ramp Drop")) -> ()
                      n71 = Subtract(x=w1261, y=w1266) -> (x-y=w1264:fxp<+/-,64,50>)
                      n72 = case shown="True" w1262 {
                        frame False {
                        }
                        frame True {
                          n73 = local write "Y Ramp Drop"(TRUE ("Start Scan")) -> ()
                          n74 = local write "Start or middle"(TRUE ("Start or middle")) -> ()
                          n75 = local write "Next Do Down Ramp"(FALSE ("Next Do Down Ramp")) -> ()
                          n76 = local write "Fly Scan"(FALSE ("Fly Scan Start")) -> ()
                        }
                      }
                      n77 = Less?(x=w1264, y=w1260) -> (x < y?=w1265:bool)
                      n78 = Select(t=w1274, s=w1272, f=u32 0) -> (s? t:f=w1270:u32)
                      n79 = local write "Continue Run"(TRUE ("Fly Scan Running")) -> ()
                      n80 = Select(t=w1260, s=w1265, f=w1264) -> (s? t:f=w1263:fxp<+/-,64,50>)
                      n81 = Select(t=u32 0, s=w1262, f=w1270) -> (s? t:f=w1276:u32)
                    }
                  }
                }
              }
              n82 = To Fixed-Point(fixed-point type=fxp<+/-,58,25> 0.0, number=w1201) -> (fixed-point=w1200:fxp<+/-,58,25>)
            }
            frame "Filtered White Noise" {
              n83 = call "White Noise Generator"("seed"=w1294, "reset"=w1292, "amplitude"=w1291) -> ("white noise out"=w1293:i16)  [unwired: 12 in]
              n84 = xnode "Butterworth Filter"("input data"=w1293, "reset"=w1292) -> ("output data"=w1289:i16)  [unwired: 1 in]
              n85 = Divide(x=w1289, y=i16 32767) -> (x/y=w1284:fxp<+/-,41,18>)
              n86 = Multiply(x=w1284, y=w1282) -> (x*y=w1287:fxp<+/-,64,35>)
              n87 = Add(x=w1287, y=w1283) -> (x+y=w1286:fxp<+/-,64,36>)
              n88 = To Fixed-Point(fixed-point type=fxp<+/-,58,25> 0.0, number=w1286) -> (fixed-point=w1285:fxp<+/-,58,25>)
            }
          }
          "X Stage Reference (nm)" <- w1167
          n89 = call "measure_loop_rate_FPGA.vi"() -> ("Loop Rate (Ticks)"=→"Measured X Reference Time Period (Ticks)":u32)  [unwired: 11 in]
          n90 = local read "stop case"() -> (w1174:bool)
          n91 = call "Loop Timer"("Count(uSec)"="X Reference Time Period (uSec)") -> ()  [unwired: 1 out]
        }
        n92 = while {
          stop <- w364 stop-if-true
          n93 = call "measure_loop_rate_FPGA.vi"() -> ("Loop Rate (Ticks)"=→"Measured Z Reference Time Period (Ticks)":u32)  [unwired: 11 in]
          n94 = call "Loop Timer10"("Count(uSec)"="Z Reference Time Period (uSec)") -> ()  [unwired: 1 out]
          n95 = case shown="\"Constant\", Default" "Z Reference Wave Selection" {
            tunnel: "Z Reference Reset" -> [_ w394 w401 w417 w450]
            tunnel: "Z Frequency (periods/tick)" -> [_ w393 w400 w416 _]
            tunnel: "Z Phase Offset (periods)" -> [_ w392 w399 w415 _]
            tunnel: "Z White Noise Seed" -> [_ _ _ _ w452]
            tunnel: "Z White Noise Amplitude" -> [_ _ _ _ w451]
            tunnel: "Z Reference DC Offset (nm)" -> [w376 w385 w396 w407 w441]
            tunnel: "Z Reference Amplitude (nm)" -> [w377 w386 w395 w409 w442]
            tunnel: [w378 w383 w397 w412 w440] -> w365
            frame "Constant", Default {
              n96 = Multiply(x=i16 1 ("y"), y=w377) -> (x*y=w381:fxp<+/-,56,33>)
              n97 = Add(x=w381, y=w376) -> (x+y=w380:fxp<+/-,56,33>)
              n98 = To Fixed-Point(fixed-point type=fxp<+/-,58,25> 0.0, number=w380) -> (fixed-point=w378:fxp<+/-,58,25>)
            }
            frame "Sine Wave" {
              n99 = call "Sine Wave Generator2"("frequency (periods/tick)"=w393, "reset"=w394, "phase offset (periods)"=w392) -> ("sine out"=w387:i16)  [unwired: 12 in]
              n100 = Divide(x=w387, y=i16 32767) -> (x/y=w390:fxp<+/-,41,18>)
              n101 = Multiply(x=w390, y=w386) -> (x*y=w389:fxp<+/-,64,35>)
              n102 = Add(x=w389, y=w385) -> (x+y=w388:fxp<+/-,64,36>)
              n103 = To Fixed-Point(fixed-point type=fxp<+/-,58,25> 0.0, number=w388) -> (fixed-point=w383:fxp<+/-,58,25>)
            }
            frame "Sawtooth Wave" {
              n104 = call "Saw Wave Generator.vi"("frequency (periods/tick)"=w400, "reset"=w401, "phase offset (periods)"=w399) -> ("saw out"=w398:i16)  [unwired: 12 in]
              n105 = Divide(x=w398, y=i16 32767) -> (x/y=w405:fxp<+/-,41,18>)
              n106 = Multiply(x=w405, y=w395) -> (x*y=w404:fxp<+/-,64,35>)
              n107 = Add(x=w404, y=w396) -> (x+y=w403:fxp<+/-,64,36>)
              n108 = To Fixed-Point(fixed-point type=fxp<+/-,58,25> 0.0, number=w403) -> (fixed-point=w397:fxp<+/-,58,25>)
            }
            frame "Square Wave" {
              w418 = fxp<+/-,32,16> 0.0 ("fixed-point type")
              n109 = call "Sine Wave Generator5"("frequency (periods/tick)"=w416, "reset"=w417, "phase offset (periods)"=w415) -> ("sine out"=w414:i16)  [unwired: 12 in]
              n110 = Divide(x=w414, y=i16 32767) -> (x/y=w438:fxp<+/-,41,18>)
              n111 = Greater?(x=w438, y=w418) -> (0:w425:bool)
              n112 = Less?(x=w438, y=w418) -> (x < y?=w424:bool)
              n113 = Equal?(x=w438, y=w418) -> (x = y?=w426:bool)
              n114 = Not(x=w425) -> (.not. x?=w422:bool)
              n115 = Not(x=w424) -> (.not. x?=w423:bool)
              n116 = Not(x=w426) -> (.not. x?=w421:bool)
              n117 = Compound Arithmetic op=AND(w425, w421, w423) -> (w427:bool)
              n118 = Compound Arithmetic op=AND(w422, w426, w423) -> (w420:bool)
              n119 = Compound Arithmetic op=AND(w422, w421, w424) -> (w419:bool)
              n120 = Select(t=fxp<+/-,2,2> 1.0 ("fixed-point type"), s=w427, f=fxp<+/-,2,2> 0.0 ("fixed-point type")) -> (s? t:f=w431:fxp<+/-,2,2>)
              n121 = Select(t=fxp<+/-,2,2> 0.0 ("fixed-point type"), s=w420, f=fxp<+/-,2,2> 0.0 ("fixed-point type")) -> (s? t:f=w430:fxp<+/-,2,2>)
              n122 = Add(x=w431, y=w430) -> (x+y=w429:fxp<+/-,3,3>)
              n123 = Select(t=fxp<+/-,2,2> -1.0 ("fixed-point type"), s=w419, f=fxp<+/-,2,2> 0.0 ("fixed-point type")) -> (s? t:f=w428:fxp<+/-,2,2>)
              n124 = Add(x=w429, y=w428) -> (x+y=w410:fxp<+/-,4,4>)
              n125 = Multiply(x=w410, y=w409) -> (x*y=w411:fxp<+/-,43,20>)
              n126 = Add(x=w411, y=w407) -> (x+y=w408:fxp<+/-,43,20>)
              n127 = To Fixed-Point(fixed-point type=fxp<+/-,58,25> 0.0, number=w408) -> (fixed-point=w412:fxp<+/-,58,25>)
            }
            frame "Filtered White Noise" {
              n128 = call "White Noise Generator3"("seed"=w452, "reset"=w450, "amplitude"=w451) -> ("white noise out"=w449:i16)  [unwired: 12 in]
              n129 = xnode "Butterworth Filter"("input data"=w449, "reset"=w450) -> ("output data"=w444:i16)  [unwired: 1 in]
              n130 = Divide(x=w444, y=i16 32767) -> (x/y=w447:fxp<+/-,41,18>)
              n131 = Multiply(x=w447, y=w442) -> (x*y=w446:fxp<+/-,64,35>)
              n132 = Add(x=w446, y=w441) -> (x+y=w445:fxp<+/-,64,36>)
              n133 = To Fixed-Point(fixed-point type=fxp<+/-,58,25> 0.0, number=w445) -> (fixed-point=w440:fxp<+/-,58,25>)
            }
          }
          "Z Stage Reference (nm)" <- w365
          n134 = local read "stop case"() -> (w364:bool)
        }
        n135 = while {
          shift-right: [w799] -> _
          shift-left: _ -> [w790]
          shift-right: [w798] -> _
          shift-left: _ -> [w789]
          shift-right: [w797] -> _
          shift-left: _ -> [w788]
          shift-right: [w796] -> _
          shift-left: _ -> [w787]
          shift-right: [w795] -> _
          shift-left: _ -> [w786]
          shift-right: [w794] -> _
          shift-left: _ -> [w785]
          shift-right: [w793] -> _
          shift-left: _ -> [w784]
          shift-right: [w792] -> _
          shift-left: _ -> [w783]
          shift-right: [w791] -> _
          shift-left: _ -> [w782]
          stop <- w811 stop-if-true
          w777 = fxp<+/-,20,5> 0.0 ("fixed-point type")
          n136 = local read "Sample X Stage Displacement (nm)"() -> (w773:fxp<+/-,58,25>)
          n137 = local read "Sample Y Stage Displacement (nm)"() -> (w770:fxp<+/-,58,25>)
          n138 = local read "Sample Z Stage Displacement (nm)"() -> (w767:fxp<+/-,58,25>)
          n139 = local read "Optics Z Stage Displacement (nm)"() -> (w766:fxp<+/-,58,25>)
          n140 = local read "Optics X Stage Displacement (nm)"() -> (w772:fxp<+/-,58,25>)
          n141 = local read "Optics Y Stage Displacement (nm)"() -> (w769:fxp<+/-,58,25>)
          n142 = case shown="\"External Reference\"" "Reference Signal Source" {
            tunnel: [w815 w818] -> w776
            tunnel: [w814 w817] -> w775
            tunnel: [w813 w816] -> w774
            frame "FPGA Generated Reference", Default {
              n143 = local read "X Stage Reference (nm)"() -> (w815:fxp<+/-,58,25>)
              n144 = local read "Y Stage Reference (nm)"() -> (w814:fxp<+/-,58,25>)
              n145 = local read "Z Stage Reference (nm)"() -> (w813:fxp<+/-,58,25>)
            }
            frame "External Reference" {
              n146 = local read "X Stage External Reference (nm)"() -> (w818:fxp<+/-,58,25>)
              n147 = local read "Y Stage External Reference (nm)"() -> (w817:fxp<+/-,58,25>)
              n148 = local read "Z Stage External Reference (nm)"() -> (w816:fxp<+/-,58,25>)
            }
          }
          n149 = call "Loop Timer3"("Count(uSec)"="Controller Time Period (uSec)") -> ()  [unwired: 1 out]
          n150 = case shown="\"Optics Stage Only\", Default" "Optics and or Sample Stage" {
            tunnel: w773 -> [_ w830]
            tunnel: w772 -> [w821 w829]
            tunnel: [w821 w828] -> w771
            tunnel: w770 -> [_ w827]
            tunnel: w769 -> [w820 w826]
            tunnel: [w820 w825] -> w768
            tunnel: w767 -> [_ w824]
            tunnel: w766 -> [w819 w823]
            tunnel: [w819 w822] -> w765
            frame "Optics Stage Only", Default {
            }
            frame "Optics and Sample Stage" {
              n151 = Subtract(x=w829, y=w830) -> (x-y=w828:fxp<+/-,59,26>)
              n152 = Subtract(x=w826, y=w827) -> (x-y=w825:fxp<+/-,59,26>)
              n153 = Subtract(x=w823, y=w824) -> (x-y=w822:fxp<+/-,59,26>)
            }
          }
          n154 = case shown="\"Closed Loop\"" "System Loop Type" {
            tunnel: w771 -> [_ w886]
            tunnel: w776 -> [w846 w887]
            tunnel: [w839 w860] -> w801
            tunnel: [w840 w885] -> w781
            tunnel: [_ w882] -> w799
            tunnel: [_ w881] -> w798
            tunnel: [_ w880] -> w797
            tunnel: [_ w879] -> w796
            tunnel: [_ w878] -> w795
            tunnel: [_ w877] -> w794
            tunnel: [_ w876] -> w793
            tunnel: [_ w875] -> w792
            tunnel: [_ w874] -> w791
            tunnel: w789 -> [_ w873]
            tunnel: w788 -> [_ w872]
            tunnel: w787 -> [_ w871]
            tunnel: w786 -> [_ w870]
            tunnel: w785 -> [_ w869]
            tunnel: w784 -> [_ w868]
            tunnel: w783 -> [_ w867]
            tunnel: w782 -> [_ w866]
            tunnel: w768 -> [_ w864]
            tunnel: w775 -> [w845 w865]
            tunnel: w774 -> [w844 w858]
            tunnel: w765 -> [_ w857]
            tunnel: [w838 w861] -> w800
            tunnel: w790 -> [_ w863]
            frame "Open Loop", Default {
              w837 = fxp<+/-,58,25> 0.0 ("fixed-point type")
              n155 = Multiply(x="X-Stage nm to V Scaling", y="X-Stage Scaling Direction") -> (x*y=w848:fxp<+/-,35,15>)
              n156 = Multiply(x="Y-Stage nm to V Scaling", y="Y-Stage Scaling Direction") -> (x*y=w834:fxp<+/-,35,15>)
              n157 = Multiply(x="Z-Stage nm to V Scaling", y="Z-Stage Scaling Direction") -> (x*y=w833:fxp<+/-,35,15>)
              n158 = Multiply(x=w846, y=w848) -> (x*y=w843:fxp<+/-,64,38>)
              n159 = Multiply(x=w845, y=w834) -> (x*y=w842:fxp<+/-,64,38>)
              n160 = Multiply(x=w844, y=w833) -> (x*y=w841:fxp<+/-,64,38>)
              n161 = To Fixed-Point(fixed-point type=w837, number=w843) -> (fixed-point=w840:fxp<+/-,58,25>)
              n162 = To Fixed-Point(fixed-point type=w837, number=w842) -> (fixed-point=w839:fxp<+/-,58,25>)
              n163 = To Fixed-Point(fixed-point type=w837, number=w841) -> (fixed-point=w838:fxp<+/-,58,25>)
            }
            frame "Closed Loop" {
              w853 = fxp<+/-,58,25> 0.0 ("fixed-point type")
              w854 = fxp<+/-,58,25> 0.0 ("fixed-point type")
              n164 = Subtract(x=w887, y=w886) -> (x-y=w891:fxp<+/-,60,27>)
              n165 = Subtract(x=w865, y=w864) -> (x-y=w890:fxp<+/-,60,27>)
              n166 = Subtract(x=w858, y=w857) -> (x-y=w859:fxp<+/-,60,27>)
              n167 = To Fixed-Point(fixed-point type=w853, number=w891) -> (fixed-point=w889:fxp<+/-,58,25>)
              n168 = To Fixed-Point(fixed-point type=w853, number=w890) -> (fixed-point=w888:fxp<+/-,58,25>)
              n169 = To Fixed-Point(fixed-point type=w853, number=w859) -> (fixed-point=w856:fxp<+/-,58,25>)
              n170 = for {
                N: 3 -> [_]
                shift-right: [w970] -> w852
                shift-left: _ -> [w968]
                shift-right: [w967] -> w851
                shift-left: _ -> [w965]
                tunnel: [w958] -> w882
                shift-right: [w957] -> _
                shift-left: _ -> [w953]
                tunnel: [w956] -> w881
                shift-right: [w955] -> _
                shift-left: _ -> [w951]
                tunnel: w863 -> [w948]
                tunnel: w873 -> [w947]
                tunnel: [w946] -> w879
                shift-right: [w945] -> _
                shift-left: _ -> [w938]
                tunnel: [w944] -> w878
                shift-right: [w943] -> _
                shift-left: _ -> [w937]
                tunnel: [w942] -> w876
                tunnel: [w941] -> w875
                shift-right: [w940] -> _
                shift-left: _ -> [w936]
                shift-right: [w939] -> _
                shift-left: _ -> [w925]
                tunnel: w871 -> [w935]
                tunnel: w870 -> [w934]
                tunnel: w868 -> [w933]
                tunnel: w867 -> [w932]
                tunnel: w889 -> [w924]
                tunnel: w888 -> [w921]
                shift-right: [w920] -> w850
                shift-left: _ -> [w917]
                tunnel: [w912] -> w880
                tunnel: [w911] -> w877
                tunnel: [w910] -> w874
                shift-right: [w909] -> _
                shift-left: _ -> [w905]
                shift-right: [w908] -> _
                shift-left: _ -> [w903]
                shift-right: [w907] -> _
                shift-left: _ -> [w901]
                tunnel: w872 -> [w900]
                tunnel: w866 -> [w899]
                tunnel: w869 -> [w898]
                tunnel: w856 -> [w894]
                i -> [w975]
                # "ez"
                # "ey"
                # "ex"
                n171 = Add(x=1, y=w975) -> (x+y=w893:i32)
                n172 = flat-sequence {
                  tunnel: [w1018] -> w985
                  tunnel: [w1017] -> w984
                  tunnel: [w1016] -> w983
                  tunnel: [w1015] -> w982
                  tunnel: [w1014] -> w981
                  tunnel: [w1013] -> w980
                  tunnel: [w1012] -> w979
                  tunnel: [w1011] -> w978
                  tunnel: w893 -> [w1019]
                  tunnel: [w997] -> w977
                  tunnel: [w1010] -> w969
                  tunnel: w968 -> [w1010]
                  tunnel: [w1009] -> w966
                  tunnel: w965 -> [w1009]
                  tunnel: [w1008] -> w954
                  tunnel: w953 -> [w1008]
                  tunnel: [w988] -> w952
                  tunnel: w951 -> [w988]
                  tunnel: w948 -> [w999]
                  tunnel: w947 -> [w1000]
                  tunnel: w938 -> [w1007]
                  tunnel: w937 -> [w1006]
                  tunnel: w936 -> [w1005]
                  tunnel: w935 -> [w1001]
                  tunnel: w934 -> [w1002]
                  tunnel: w933 -> [w1003]
                  tunnel: w932 -> [w1004]
                  tunnel: w925 -> [w998]
                  tunnel: [w1007] -> w931
                  tunnel: [w1006] -> w930
                  tunnel: [w1005] -> w929
                  tunnel: w924 -> [w987]
                  tunnel: [w998] -> w923
                  tunnel: w921 -> [w986]
                  tunnel: [w996] -> w918
                  tunnel: w917 -> [w996]
                  tunnel: [w995] -> w906
                  tunnel: w905 -> [w995]
                  tunnel: [w994] -> w904
                  tunnel: w903 -> [w994]
                  tunnel: [w993] -> w902
                  tunnel: w901 -> [w993]
                  tunnel: w900 -> [w990]
                  tunnel: w899 -> [w992]
                  tunnel: w898 -> [w991]
                  tunnel: w894 -> [w989]
                  tunnel: w985 -> [w1071]
                  tunnel: w984 -> [w1070]
                  tunnel: w983 -> [w1069]
                  tunnel: w982 -> [w1049]
                  tunnel: w981 -> [w1050]
                  tunnel: w980 -> [w1051]
                  tunnel: w979 -> [w1052]
                  tunnel: w978 -> [w1053]
                  tunnel: w977 -> [w1058]
                  tunnel: [w1056] -> w974
                  tunnel: [w1056] -> w973
                  tunnel: [w1047] -> w972
                  tunnel: [w1048] -> w971
                  tunnel: w969 -> [w1048]
                  tunnel: w966 -> [w1047]
                  tunnel: [w1057] -> w964
                  tunnel: [w1057] -> w963
                  tunnel: [w1055] -> w962
                  tunnel: [w1055] -> w961
                  tunnel: [w1054] -> w960
                  tunnel: [w1054] -> w959
                  tunnel: w954 -> [w1068]
                  tunnel: w952 -> [w1067]
                  tunnel: [w1068] -> w950
                  tunnel: [w1067] -> w949
                  tunnel: w931 -> [w1066]
                  tunnel: w930 -> [w1065]
                  tunnel: w929 -> [w1064]
                  tunnel: [w1066] -> w928
                  tunnel: [w1065] -> w927
                  tunnel: [w1064] -> w926
                  tunnel: w923 -> [w1063]
                  tunnel: [w1063] -> w922
                  tunnel: [w1056] -> w919
                  tunnel: w918 -> [w1062]
                  tunnel: [w1062] -> w916
                  tunnel: [w1057] -> w915
                  tunnel: [w1055] -> w914
                  tunnel: [w1054] -> w913
                  tunnel: w906 -> [w1061]
                  tunnel: w904 -> [w1060]
                  tunnel: w902 -> [w1059]
                  tunnel: [w1061] -> w897
                  tunnel: [w1060] -> w896
                  tunnel: [w1059] -> w895
                  tunnel: w974 -> [w1099]
                  tunnel: w973 -> [w1154]
                  tunnel: w893 -> [w1098]
                  tunnel: w972 -> [w1153]
                  tunnel: w971 -> [w1100]
                  tunnel: [w1103] -> w970
                  tunnel: [w1102] -> w967
                  tunnel: w964 -> [w1140]
                  tunnel: w963 -> [w1139]
                  tunnel: w962 -> [w1138]
                  tunnel: w961 -> [w1137]
                  tunnel: w960 -> [w1136]
                  tunnel: w959 -> [w1135]
                  tunnel: [w1134] -> w958
                  tunnel: [w1134] -> w957
                  tunnel: [w1133] -> w956
                  tunnel: [w1133] -> w955
                  tunnel: w950 -> [w1132]
                  tunnel: w949 -> [w1131]
                  tunnel: [w1130] -> w946
                  tunnel: [w1130] -> w945
                  tunnel: [w1129] -> w944
                  tunnel: [w1129] -> w943
                  tunnel: [w1128] -> w942
                  tunnel: [w1127] -> w941
                  tunnel: [w1128] -> w940
                  tunnel: [w1127] -> w939
                  tunnel: w928 -> [w1126]
                  tunnel: w927 -> [w1125]
                  tunnel: w926 -> [w1124]
                  tunnel: w922 -> [w1123]
                  tunnel: [w1101] -> w920
                  tunnel: w919 -> [w1120]
                  tunnel: w916 -> [w1119]
                  tunnel: w915 -> [w1112]
                  tunnel: w914 -> [w1111]
                  tunnel: w913 -> [w1110]
                  tunnel: [w1109] -> w912
                  tunnel: [w1108] -> w911
                  tunnel: [w1107] -> w910
                  tunnel: [w1109] -> w909
                  tunnel: [w1108] -> w908
                  tunnel: [w1107] -> w907
                  tunnel: w897 -> [w1106]
                  tunnel: w896 -> [w1105]
                  tunnel: w895 -> [w1104]
                  frame #0 {
                    n173 = case shown="1, Default" w1019 {
                      tunnel: ["sos gain SF Controller xx1" "sos gain SF Controller yy1" "sos gain SF Controller zz1"] -> w1015
                      tunnel: ["-a01(2) xx1" "-a01(2) yy1" "-a01(2) zz1"] -> w1014
                      tunnel: ["-a02(2) xx1" "-a02(2) yy1" "-a02(2) zz1"] -> w1013
                      tunnel: ["b01(2) xx1" "b01(2) yy1" "b01(2) zz1"] -> w1012
                      tunnel: ["b02(2) xx1" "b02(2) yy1" "b02(2) zz1"] -> w1011
                      tunnel: [w1020 w1031 w1045] -> w1016
                      tunnel: [w1026 w1030 w1044] -> w1017
                      tunnel: [w1027 w1029 w1043] -> w1018
                      tunnel: w999 -> [w1027 _ _]
                      tunnel: w1000 -> [_ w1029 _]
                      tunnel: w1001 -> [w1026 _ _]
                      tunnel: w1002 -> [_ w1030 _]
                      tunnel: w1003 -> [w1020 _ _]
                      tunnel: w1004 -> [_ w1031 _]
                      tunnel: [w1028 w1037 w1046] -> w997
                      tunnel: w987 -> [w1028 _ _]
                      tunnel: w986 -> [_ w1037 _]
                      tunnel: w992 -> [_ _ w1045]
                      tunnel: w991 -> [_ _ w1044]
                      tunnel: w990 -> [_ _ w1043]
                      tunnel: w989 -> [_ _ w1046]
                      frame 1, Default {
                      }
                      frame 2 {
                      }
                      frame 3 {
                      }
                    }
                  }
                  frame #1 {
                    # "n_i"
                    # "m_i"
                    # "l_i"
                    # "u_i"
                    n174 = Multiply(x=w1058, y=w1049) -> (x*y=w1072:fxp<+/-,64,34>)
                    n175 = To Fixed-Point(number=w1072) -> (fixed-point=w1073:fxp<+/-,58,25>)  [unwired: 1 in]
                    n176 = for {
                      tunnel: w1050 -> [w1089] mode=indexing
                      tunnel: w1053 -> [w1086] mode=indexing
                      shift-right: [w1091] -> w1056
                      shift-left: w1073 -> [w1090]
                      tunnel: w1051 -> [w1088] mode=indexing
                      tunnel: w1052 -> [w1087] mode=indexing
                      tunnel: [w1078] -> w1057 mode=indexing
                      tunnel: w1071 -> [w1084] mode=indexing
                      tunnel: [w1081] -> w1055 mode=indexing
                      tunnel: w1070 -> [w1074] mode=indexing
                      tunnel: [w1074] -> w1054 mode=indexing
                      tunnel: w1069 -> [w1082] mode=indexing
                      # "b_1"
                      # "b_2"
                      # "n_i-1"
                      # "-a_2"
                      # "-a_1"
                      # "m_i-1"
                      # "l_i-1"
                      # "e_i"
                      n177 = To Fixed-Point(number=w1084) -> (fixed-point=w1097:fxp<+/-,58,25>)  [unwired: 1 in]
                      n178 = Add(x=w1090, y=w1097) -> (x+y=w1083:fxp<+/-,59,26>)
                      n179 = To Fixed-Point(number=w1083) -> (fixed-point=w1081:fxp<+/-,58,25>)  [unwired: 1 in]
                      n180 = Multiply(x=w1081, y=w1089) -> (x*y=w1096:fxp<+/-,64,34>)
                      n181 = Multiply(x=w1082, y=w1086) -> (x*y=w1095:fxp<+/-,64,34>)
                      n182 = Multiply(x=w1074, y=w1088) -> (x*y=w1092:fxp<+/-,64,34>)
                      n183 = To Fixed-Point(number=w1096) -> (fixed-point=w1077:fxp<+/-,58,25>)  [unwired: 1 in]
                      n184 = To Fixed-Point(number=w1092) -> (fixed-point=w1076:fxp<+/-,58,25>)  [unwired: 1 in]
                      n185 = To Fixed-Point(number=w1095) -> (fixed-point=w1075:fxp<+/-,58,25>)  [unwired: 1 in]
                      n186 = Add(x=w1077, y=w1076) -> (x+y=w1085:fxp<+/-,59,26>)
                      n187 = To Fixed-Point(number=w1085) -> (fixed-point=w1078:fxp<+/-,58,25>)  [unwired: 1 in]
                      n188 = Multiply(x=w1074, y=w1087) -> (x*y=w1093:fxp<+/-,64,34>)
                      n189 = To Fixed-Point(number=w1093) -> (fixed-point=w1079:fxp<+/-,58,25>)  [unwired: 1 in]
                      n190 = Add(x=w1079, y=w1075) -> (x+y=w1094:fxp<+/-,59,26>)
                      n191 = To Fixed-Point(number=w1094) -> (fixed-point=w1080:fxp<+/-,58,25>)  [unwired: 1 in]
                      n192 = Add(x=w1081, y=w1080) -> (x+y=w1091:fxp<+/-,58,25>)
                    }
                  }
                  frame #2 {
                    n193 = Equal?(x=3, y=w1098) -> (x = y?=w1121:bool)
                    n194 = Equal?(x=2, y=w1098) -> (x = y?=w1155:bool)
                    n195 = Equal?(x=1, y=w1098) -> (x = y?=w1157:bool)
                    n196 = Equal?(x=2, y=w1098) -> (x = y?=w1145:bool)
                    n197 = Equal?(x=2, y=w1098) -> (x = y?=w1149:bool)
                    n198 = Equal?(x=3, y=w1098) -> (x = y?=w1117:bool)
                    n199 = Equal?(x=2, y=w1098) -> (x = y?=w1141:bool)
                    n200 = Equal?(x=1, y=w1098) -> (x = y?=w1151:bool)
                    n201 = Equal?(x=1, y=w1098) -> (x = y?=w1147:bool)
                    n202 = Equal?(x=3, y=w1098) -> (x = y?=w1115:bool)
                    n203 = Equal?(x=1, y=w1098) -> (x = y?=w1143:bool)
                    n204 = Equal?(x=3, y=w1098) -> (x = y?=w1113:bool)
                    n205 = Select(t=w1120, s=w1121, f=w1119) -> (s? t:f=w1101:fxp<+/-,58,25>)
                    "Kzz Output, Kzz*ez (V)" <- w1101
                    n206 = Select(t=w1154, s=w1155, f=w1153) -> (s? t:f=w1102:fxp<+/-,58,25>)
                    "Kyy Output, Kyy*ey (V)" <- w1102
                    n207 = Select(t=w1099, s=w1157, f=w1100) -> (s? t:f=w1103:fxp<+/-,58,25>)
                    "Kxx Output, Kxx*ex (V)" <- w1103
                    n208 = Select(t=w1137, s=w1145, f=w1125) -> (s? t:f=w1129:fxp<+/-,58,25>[])
                    n209 = Select(t=w1139, s=w1149, f=w1131) -> (s? t:f=w1133:fxp<+/-,58,25>[])
                    n210 = Select(t=w1112, s=w1117, f=w1106) -> (s? t:f=w1109:fxp<+/-,58,25>[])
                    n211 = Select(t=w1135, s=w1141, f=w1123) -> (s? t:f=w1127:fxp<+/-,58,25>[])
                    n212 = Select(t=w1140, s=w1151, f=w1132) -> (s? t:f=w1134:fxp<+/-,58,25>[])
                    n213 = Select(t=w1138, s=w1147, f=w1126) -> (s? t:f=w1130:fxp<+/-,58,25>[])
                    n214 = Select(t=w1111, s=w1115, f=w1105) -> (s? t:f=w1108:fxp<+/-,58,25>[])
                    n215 = Select(t=w1136, s=w1143, f=w1124) -> (s? t:f=w1128:fxp<+/-,58,25>[])
                    n216 = Select(t=w1110, s=w1113, f=w1104) -> (s? t:f=w1107:fxp<+/-,58,25>[])
                  }
                }
              }
              n217 = Multiply(x=w850, y="Scaling mV to V") -> (x*y=w884:fxp<+/-,64,35>)
              n218 = Multiply(x=w852, y="Scaling mV to V") -> (x*y=w883:fxp<+/-,64,35>)
              n219 = Multiply(x=w851, y="Scaling mV to V") -> (x*y=w862:fxp<+/-,64,35>)
              n220 = To Fixed-Point(fixed-point type=w854, number=w883) -> (fixed-point=w885:fxp<+/-,58,25>)
              n221 = To Fixed-Point(fixed-point type=w854, number=w862) -> (fixed-point=w860:fxp<+/-,58,25>)
              n222 = To Fixed-Point(fixed-point type=w854, number=w884) -> (fixed-point=w861:fxp<+/-,58,25>)
            }
          }
          n223 = local read "stop case"() -> (w811:bool)
          n224 = To Fixed-Point(fixed-point type=w777, number=w781) -> (fixed-point=w780:fxp<+/-,20,5>)
          n225 = To Fixed-Point(fixed-point type=w777, number=w801) -> (fixed-point=w779:fxp<+/-,20,5>)
          n226 = To Fixed-Point(fixed-point type=w777, number=w800) -> (fixed-point=w778:fxp<+/-,20,5>)
          n227 = call "measure_loop_rate_FPGA.vi"() -> ("Loop Rate (Ticks)"=→"Measured Controller Time Period (Ticks)":u32)  [unwired: 11 in]
          n228 = In Range and Coerce(upper limit="Controller Output Upper Limit", x=w780, lower limit="Controller Output Lower Limit") -> (coerced(x)=→"PI X-Stage Input (V)":fxp<+/-,20,5>, In Range?=→"X-Stage Input In Range?":bool)
          n229 = In Range and Coerce(upper limit="Controller Output Upper Limit", x=w779, lower limit="Controller Output Lower Limit") -> (coerced(x)=→"PI Y-Stage Input (V)":fxp<+/-,20,5>, In Range?=→"Y-Stage Input In Range?":bool)
          n230 = In Range and Coerce(upper limit="Controller Output Upper Limit", x=w778, lower limit="Controller Output Lower Limit") -> (coerced(x)=→"PI Z-Stage Input (V)":fxp<+/-,20,5>, In Range?=→"Z-Stage Input In Range?":bool)
        }
        n231 = while {
          shift-right: [w620] -> _
          shift-left: i16 0 -> [w619]
          shift-right: [w618] -> _
          shift-left: i16 0 -> [w617]
          stop <- w630 stop-if-true
          n232 = local read "Fly Scan Running"() -> (w609:bool)
          n233 = case shown="\"Square Wave 1\"" "Trigger Wave Generator" {
            tunnel: [w646 w690 w712] -> w621
            tunnel: [w644 _ _] -> w620
            tunnel: w619 -> [w643 _ _]
            tunnel: [w637 _ _] -> w618
            tunnel: w617 -> [w636 _ _]
            tunnel: "DT Reset" -> [_ w696 w717]
            tunnel: "DT Frequency (periods/tick)" -> [_ w695 w716]
            tunnel: "DT Phase Offset (periods)" -> [_ w694 w715]
            tunnel: "DT Duty Cycle (periods)" -> [_ w693 _]
            tunnel: "DT Reference Amplitude (V)" -> [_ w692 w714]
            tunnel: "DT Reference DC Offset (V)" -> [_ w691 w713]
            tunnel: w609 -> [w631 w689 w711]
            frame "Custom Square Wave ", Default {
              n234 = local read "If True End Trigger High"() -> (w635:bool)
              n235 = local read "If True End Trigger Low"() -> (w634:bool)
              n236 = Not(x=w635) -> (.not. x?=w633:bool)
              n237 = Compound Arithmetic op=AND(w634, w633) -> (w632:bool)
              n238 = local read "Trigger Generation Time Period (uSec)"() -> (w642:u32)
              n239 = case shown="True" w632 {
                tunnel: [Detector_Trigger_Control."Trigger Low" Detector_Trigger_Control."Trigger High"] -> w645
                frame False {
                }
                frame True {
                }
              }
              n240 = case shown="True" w631 {
                tunnel: [fxp<+/-,20,5> 0.0 ("Trigger High Level (V)") w652] -> w646
                tunnel: w645 -> [_ w660]
                tunnel: [_ w659] -> w644
                tunnel: w643 -> [_ w658]
                tunnel: w642 -> [_ w657]
                tunnel: "Trigger High Period (usec)" -> [_ w656]
                tunnel: "Trigger Low Period (usec)" -> [_ w655]
                tunnel: "Trigger High Level (V)" -> [_ w654]
                tunnel: "Trigger Low Level (V)" -> [_ w653]
                tunnel: [_ w651] -> w637
                tunnel: w636 -> [_ w650]
                frame False {
                  n241 = local write "If True End Trigger High"(FALSE ("If True End Trigger High")) -> ()
                  n242 = local write "If True End Trigger Low"(TRUE ("If True End Trigger Low")) -> ()
                }
                frame True {
                  n243 = case shown="\"Trigger High\", Default" w660 {
                    tunnel: [w671 _] -> w659
                    tunnel: w658 -> [w670 _]
                    tunnel: w657 -> [w667 w681]
                    tunnel: w656 -> [w665 _]
                    tunnel: w655 -> [_ w679]
                    tunnel: w654 -> [w662 _]
                    tunnel: w653 -> [_ w674]
                    tunnel: [w662 w674] -> w652
                    tunnel: [_ w684] -> w651
                    tunnel: w650 -> [_ w683]
                    frame "Trigger High", Default {
                      n244 = Increment(x=w670) -> (x+1=w668:i16)
                      n245 = Multiply(x=w668, y=w667) -> (x*y=w666:u32)
                      n246 = Less Or Equal?(x=w666, y=w665) -> (x <= y?=w664:bool)
                      "Trigger Mid High" <- w664
                      n247 = Greater?(x=w666, y=w665) -> (0:w661:bool)
                      "If True End Trigger High" <- w661
                      n248 = case shown="True" w661 {
                        frame False {
                        }
                        frame True {
                          n249 = local write "If True End Trigger Low"(FALSE) -> ()
                        }
                      }
                      n250 = Select(t=w668, s=w664, f=i16 0) -> (s? t:f=w669:i16)
                      n251 = Select(t=i16 0, s=w661, f=w669) -> (s? t:f=w671:i16)
                    }
                    frame "Trigger Low" {
                      n252 = Increment(x=w683) -> (x+1=w682:i16)
                      n253 = Multiply(x=w682, y=w681) -> (x*y=w680:u32)
                      n254 = Less Or Equal?(x=w680, y=w679) -> (x <= y?=w678:bool)
                      n255 = Greater?(x=w680, y=w679) -> (0:w675:bool)
                      "If True End Trigger Low" <- w675
                      n256 = case shown="True" w675 {
                        frame False {
                        }
                        frame True {
                          n257 = local write "If True End Trigger High"(FALSE) -> ()
                        }
                      }
                      n258 = Select(t=w682, s=w678, f=i16 0) -> (s? t:f=w676:i16)
                      n259 = Select(t=i16 0, s=w675, f=w676) -> (s? t:f=w684:i16)
                    }
                  }
                }
              }
            }
            frame "Square Wave 1" {
              n260 = case shown="True" w689 {
                tunnel: w696 -> [_ w704]
                tunnel: w695 -> [_ w703]
                tunnel: w694 -> [_ w702]
                tunnel: w693 -> [_ w701]
                tunnel: w692 -> [_ w700]
                tunnel: w691 -> [_ w699]
                tunnel: [fxp<+/-,58,25> 0.0 ("fixed-point type") w698] -> w690
                frame False {
                }
                frame True {
                  n261 = call "Square Wave Generator"("frequency (periods/tick)"=w703, "reset"=w704, "phase offset (periods)"=w702, "duty cycle (periods)"=w701) -> ("square wave out"=w710:i16)  [unwired: 11 in]
                  n262 = Divide(x=w710, y=i16 32767) -> (x/y=w708:fxp<+/-,41,18>)
                  n263 = Multiply(x=w708, y=w700) -> (x*y=w707:fxp<+/-,64,35>)
                  n264 = Add(x=w707, y=w699) -> (x+y=w706:fxp<+/-,64,36>)
                  n265 = To Fixed-Point(fixed-point type=fxp<+/-,58,25> 0.0, number=w706) -> (fixed-point=w698:fxp<+/-,58,25>)
                }
              }
            }
            frame "Square Wave 2" {
              n266 = case shown="False" w711 {
                tunnel: w716 -> [_ w724]
                tunnel: w715 -> [_ w723]
                tunnel: w717 -> [_ w722]
                tunnel: w714 -> [_ w721]
                tunnel: w713 -> [_ w720]
                tunnel: [fxp<+/-,58,25> 0.0 ("fixed-point type") w719] -> w712
                frame False {
                }
                frame True {
                  w730 = fxp<+/-,32,16> 0.0 ("fixed-point type")
                  n267 = call "Sine Wave Generator3"("frequency (periods/tick)"=w724, "reset"=w722, "phase offset (periods)"=w723) -> ("sine out"=w729:i16)  [unwired: 12 in]
                  n268 = Divide(x=w729, y=i16 32767) -> (x/y=w750:fxp<+/-,41,18>)
                  n269 = Greater?(x=w750, y=w730) -> (0:w737:bool)
                  n270 = Equal?(x=w750, y=w730) -> (x = y?=w738:bool)
                  n271 = Less?(x=w750, y=w730) -> (x < y?=w736:bool)
                  n272 = Not(x=w737) -> (.not. x?=w734:bool)
                  n273 = Not(x=w738) -> (.not. x?=w733:bool)
                  n274 = Not(x=w736) -> (.not. x?=w735:bool)
                  n275 = Compound Arithmetic op=AND(w737, w733, w735) -> (w739:bool)
                  n276 = Compound Arithmetic op=AND(w734, w738, w735) -> (w732:bool)
                  n277 = Compound Arithmetic op=AND(w734, w733, w736) -> (w731:bool)
                  n278 = Select(t=fxp<+/-,2,2> 1.0 ("fixed-point type"), s=w739, f=fxp<+/-,2,2> 0.0 ("fixed-point type")) -> (s? t:f=w743:fxp<+/-,2,2>)
                  n279 = Select(t=fxp<+/-,2,2> 0.0 ("fixed-point type"), s=w732, f=fxp<+/-,2,2> 0.0 ("fixed-point type")) -> (s? t:f=w742:fxp<+/-,2,2>)
                  n280 = Select(t=fxp<+/-,2,2> -1.0 ("fixed-point type"), s=w731, f=fxp<+/-,2,2> 0.0 ("fixed-point type")) -> (s? t:f=w740:fxp<+/-,2,2>)
                  n281 = Add(x=w743, y=w742) -> (x+y=w741:fxp<+/-,3,3>)
                  n282 = Add(x=w741, y=w740) -> (x+y=w726:fxp<+/-,4,4>)
                  n283 = Multiply(x=w726, y=w721) -> (x*y=w727:fxp<+/-,43,20>)
                  n284 = Add(x=w727, y=w720) -> (x+y=w725:fxp<+/-,43,20>)
                  n285 = To Fixed-Point(fixed-point type=fxp<+/-,58,25> 0.0, number=w725) -> (fixed-point=w719:fxp<+/-,58,25>)
                }
              }
            }
          }
          n286 = call "measure_loop_rate_FPGA.vi"() -> ("Loop Rate (Ticks)"=→"Measured Trigger Gen Time Period (Ticks)":u32)  [unwired: 11 in]
          n287 = To Fixed-Point(fixed-point type=fxp<+/-,20,5> 0.0, number=w621) -> (fixed-point=w622:fxp<+/-,20,5>)
          n288 = In Range and Coerce(upper limit="Detector Trigger Upper Limit (V)", x=w622, lower limit="Detector Trigger Lower Limit (V)") -> (coerced(x)=→"Detector Trigger (V)":fxp<+/-,20,5>, In Range?=→"Detector Trigger In Range?":bool)
          n289 = call "Loop Timer7"("Count(uSec)"="Trigger Generation Time Period (uSec)") -> ()  [unwired: 1 out]
          n290 = local read "stop case"() -> (w630:bool)
        }
        n291 = while {
          tunnel: [w754] -> w70
          stop <- w760 stop-if-true
          n292 = local read "Detector Trigger (V)"() -> (w753:fxp<+/-,20,5>)
          n293 = local read "PI X-Stage Input (V)"() -> (w757:fxp<+/-,20,5>)
          n294 = local read "PI Y-Stage Input (V)"() -> (w756:fxp<+/-,20,5>)
          n295 = local read "PI Z-Stage Input (V)"() -> (w755:fxp<+/-,20,5>)
          n296 = xnode "FPGA I/O Node"("Mod8/AO0"=w757, "Mod8/AO1"=w756, "Mod8/AO2"=w755, "Mod8/AO3"=w753) -> ("error out"=w754:errorcluster)  [unwired: 5 in, 4 out]
          n297 = call "Loop Timer4"("Count(uSec)"="Controller Output Time Period (uSec)") -> ()  [unwired: 1 out]
          n298 = call "measure_loop_rate_FPGA.vi"() -> ("Loop Rate (Ticks)"=→"Measured Controller Output Time Period (Ticks)" →"Measured Detector Trigger Time Period (Ticks)":u32)  [unwired: 11 in]
          n299 = local read "stop case"() -> (w759:bool)
          n300 = Unbundle By Name(w754) -> ("status"=w758:bool)
          n301 = Or(x=w758, y=w759) -> (x .or. y?=w760:bool)
        }
        n302 = while {
          shift-right: [w469] -> _
          shift-left: w69 -> [w464]
          shift-right: [w468] -> _
          shift-left: u32 0 ("f") -> [w466]
          shift-right: [w467] -> _
          shift-left: u32 0 -> [w465]
          tunnel: w69 -> [w461]
          stop <- w470 stop-if-true
          n303 = case shown="\"Custom Ramp Wave\"" "Y Reference Wave Selection" {
            tunnel: "Y Reference Amplitude (nm)" -> [w487 w491 _ w592]
            tunnel: "Y Reference DC Offset (nm)" -> [w486 w490 _ w591]
            tunnel: [w482 w489 w517 w588] -> w478
            tunnel: "Y Frequency (periods/tick)" -> [_ w500 _ _]
            tunnel: "Y Phase Offset (periods)" -> [_ w499 _ _]
            tunnel: "Y Reference Reset" -> [_ w498 _ w597]
            tunnel: "Y White Noise Seed" -> [_ _ _ w600]
            tunnel: "Y White Noise Amplitude" -> [_ _ _ w599]
            tunnel: [_ _ w515 _] -> w469
            tunnel: [_ _ w513 _] -> w468
            tunnel: [_ _ w512 _] -> w467
            tunnel: w466 -> [_ _ w511 _]
            tunnel: w465 -> [_ _ w510 _]
            tunnel: w464 -> [_ _ w508 _]
            tunnel: "Y Ramp Period (usec)" -> [_ _ w504 _]
            tunnel: "Y Ramp End (nm)" -> [_ _ w503 _]
            tunnel: w461 -> [_ _ w502 _]
            frame "Constant", Default {
              n304 = Multiply(x=i16 1 ("y"), y=w487) -> (x*y=w485:fxp<+/-,56,33>)
              n305 = Add(x=w485, y=w486) -> (x+y=w484:fxp<+/-,56,33>)
              n306 = To Fixed-Point(fixed-point type=fxp<+/-,58,25> 0.0, number=w484) -> (fixed-point=w482:fxp<+/-,58,25>)
            }
            frame "Sine Wave" {
              n307 = call "Sine Wave Generator4"("frequency (periods/tick)"=w500, "reset"=w498, "phase offset (periods)"=w499) -> ("sine out"=w497:i16)  [unwired: 12 in]
              n308 = Divide(x=w497, y=i16 32767) -> (x/y=w495:fxp<+/-,41,18>)
              n309 = Multiply(x=w495, y=w491) -> (x*y=w494:fxp<+/-,64,35>)
              n310 = Add(x=w494, y=w490) -> (x+y=w493:fxp<+/-,64,36>)
              n311 = To Fixed-Point(fixed-point type=fxp<+/-,58,25> 0.0, number=w493) -> (fixed-point=w489:fxp<+/-,58,25>)
            }
            frame "Custom Ramp Wave" {
              n312 = Subtract(x=w502, y=w503) -> (x-y=w522:fxp<+/-,17,17>)
              n313 = Less?(x=w502, y=w503) -> (x < y?=w507:bool)
              n314 = Absolute Value(x=w522) -> (abs(x)=w521:fxp<+,16,16>)
              n315 = local read "Continue Run"() -> (w506:bool)
              n316 = Divide(x=w521, y=w504) -> (x/y=w523:fxp<+,48,16>)
              "Y Ramp Slope" <- w523
              n317 = local read "Start or middle"() -> (w519:bool)
              n318 = local read "Y Reference Time Period (uSec)"() -> (w509:u32)
              n319 = case shown="False" w507 {
                tunnel: [Control_Y_Up_Down_Ramp."Y Down Ramp" Control_Y_Up_Down_Ramp."Y Up Ramp"] -> w505
                frame False {
                }
                frame True {
                }
              }
              n320 = Compound Arithmetic op=OR("Fly Scan", w506) -> (w514:bool)
              "Fly Scan Running" <- w514
              n321 = Select(t=w508, s=w519, f=w502) -> (s? t:f=w520:fxp<+/-,58,25>)
              n322 = case shown="True" w514 {
                tunnel: w505 -> [_ w541]
                tunnel: w509 -> [_ w540]
                tunnel: ["Y Start Marker (nm)" w539] -> w518
                tunnel: w504 -> [_ w538]
                tunnel: w523 -> [_ w537]
                tunnel: w502 -> [_ w536]
                tunnel: w503 -> [_ w535]
                tunnel: [_ w534] -> w513
                tunnel: [_ w533] -> w512
                tunnel: w511 -> [_ w532]
                tunnel: w510 -> [_ w531]
                tunnel: [_ w530] -> w515
                tunnel: w520 -> [_ w529]
                frame False {
                  "Start or middle" <- FALSE ("Start or middle")
                  "Y scan done" <- TRUE
                }
                frame True {
                  n323 = case shown="\"Y Down Ramp\"" w541 {
                    tunnel: [w560 _] -> w534
                    tunnel: w532 -> [w559 _]
                    tunnel: w540 -> [w556 w577]
                    tunnel: w538 -> [w555 w573]
                    tunnel: w536 -> [w545 _]
                    tunnel: w535 -> [w549 w566]
                    tunnel: [_ w580] -> w533
                    tunnel: w531 -> [_ w579]
                    tunnel: w537 -> [w551 _]
                    tunnel: [w543 w562] -> w539
                    tunnel: [_ w562] -> w530
                    tunnel: w529 -> [_ w564]
                    frame "Y Up Ramp", Default {
                      n324 = Increment(x=w559) -> (x+1=w557:u32)
                      n325 = Multiply(x=w557, y=w556) -> (x*y=w552:u32)
                      n326 = Multiply(x=w552, y=w551) -> (x*y=w550:fxp<+,64,48>)
                      n327 = Less Or Equal?(x=w552, y=w555) -> (x <= y?=w554:bool)
                      "Ramp Mid Range" <- w554
                      n328 = Add(x=w550, y=w545) -> (x+y=w548:fxp<+/-,64,50>)
                      n329 = Greater?(x=w552, y=w555) -> (0:w544:bool)
                      "If True End Up Ramp" <- w544
                      n330 = Greater?(x=w548, y=w549) -> (0:w546:bool)
                      n331 = Select(t=w557, s=w554, f=i16 0) -> (s? t:f=w558:u32)
                      n332 = Select(t=w545, s=w546, f=w548) -> (s? t:f=w547:fxp<+/-,64,50>)
                      n333 = Select(t=i16 0, s=w544, f=w558) -> (s? t:f=w560:u32)
                      n334 = To Fixed-Point(fixed-point type=fxp<+/-,58,25> 0.0, number=w547) -> (fixed-point=w543:fxp<+/-,58,25>)
                    }
                    frame "Y Down Ramp" {
                      n335 = Increment(x=w579) -> (x+1=w578:u32)
                      n336 = local read "Y Ramp Drop"() -> (w570:bool)
                      n337 = Multiply(x=w578, y=w577) -> (x*y=w572:u32)
                      n338 = Less Or Equal?(x=w572, y=w573) -> (x <= y?=w576:bool)
                      n339 = Greater?(x=w572, y=w573) -> (0:w571:bool)
                      "If True End Y Down Ramp" <- w571
                      n340 = case shown="True" w570 {
                        tunnel: "Y Ramp Drop Size (nm)" -> [_ w585]
                        tunnel: [w582 w584] -> w568
                        tunnel: w564 -> [w582 w583]
                        frame False {
                        }
                        frame True {
                          n341 = Subtract(x=w583, y=w585) -> (x-y=w584:fxp<+/-,59,26>)
                        }
                      }
                      n342 = Select(t=w578, s=w576, f=u32 0) -> (s? t:f=w574:u32)
                      n343 = To Fixed-Point(fixed-point type=fxp<+/-,58,25> 0.0, number=w568) -> (fixed-point=w563:fxp<+/-,58,25>)
                      n344 = Less?(x=w563, y=w566) -> (x < y?=w565:bool)
                      n345 = case shown="True" w565 {
                        frame False {
                        }
                        frame True {
                          n346 = local write "Fly Scan Running"(FALSE ("Fly Scan Running")) -> ()
                          n347 = local write "Continue Run"(FALSE ("Start Scan")) -> ()
                        }
                      }
                      n348 = Select(t=u32 0, s=w571, f=w574) -> (s? t:f=w580:u32)
                      n349 = Select(t=w564, s=w565, f=w563) -> (s? t:f=w562:fxp<+/-,58,25>)
                    }
                  }
                }
              }
              n350 = To Fixed-Point(fixed-point type=fxp<+/-,58,25> 0.0, number=w518) -> (fixed-point=w517:fxp<+/-,58,25>)
            }
            frame "Filtered White Noise" {
              n351 = call "White Noise Generator2"("seed"=w600, "reset"=w597, "amplitude"=w599) -> ("white noise out"=w598:i16)  [unwired: 12 in]
              n352 = xnode "Butterworth Filter"("input data"=w598, "reset"=w597) -> ("output data"=w595:i16)  [unwired: 1 in]
              n353 = Divide(x=w595, y=i16 32767) -> (x/y=w594:fxp<+/-,41,18>)
              n354 = Multiply(x=w594, y=w592) -> (x*y=w593:fxp<+/-,64,35>)
              n355 = Add(x=w593, y=w591) -> (x+y=w590:fxp<+/-,64,36>)
              n356 = To Fixed-Point(fixed-point type=fxp<+/-,58,25> 0.0, number=w590) -> (fixed-point=w588:fxp<+/-,58,25>)
            }
          }
          "Y Stage Reference (nm)" <- w478
          n357 = call "measure_loop_rate_FPGA.vi"() -> ("Loop Rate (Ticks)"=→"Measured Y Reference Time Period (Ticks)":u32)  [unwired: 11 in]
          n358 = local read "stop case"() -> (w470:bool)
          n359 = call "Loop Timer9"("Count(uSec)"="Y Reference Time Period (uSec)") -> ()  [unwired: 1 out]
        }
        n360 = case shown="\"Fly\", Default" "Scan type" {
          tunnel: [w105 errorcluster {"Status?"=FALSE, "Code"=0, "Source"=""} ("error out")] -> w81
          frame "Fly", Default {
            n361 = while {
              tunnel: [w118] -> w105
              shift-right: [w106] -> _
              shift-left: _ -> [w111]
              stop <- w116 stop-if-true
              n362 = local read "Detector Trigger (V)"() -> (w106:fxp<+/-,20,5>)
              n363 = call "Loop Timer2"("Count(uSec)"="Datalog Time Period (uSec)") -> ()  [unwired: 1 out]
              n364 = Greater?(x=w106, y=w111) -> (0:w110:bool)
              n365 = case shown="True" w110 {
                tunnel: [_ w127] -> w119
                tunnel: [_ w123] -> w112
                frame False {
                }
                frame True {
                  w128 = 5  # # of Data Strings
                  n366 = local read "Sample X Stage Displacement (nm)"() -> (w134:fxp<+/-,58,25>)
                  n367 = local read "Sample Y Stage Displacement (nm)"() -> (w133:fxp<+/-,58,25>)
                  n368 = local read "Sample Z Stage Displacement (nm)"() -> (w132:fxp<+/-,58,25>)
                  n369 = local read "Optics X Stage Displacement (nm)"() -> (w138:fxp<+/-,58,25>)
                  n370 = local read "Optics Y Stage Displacement (nm)"() -> (w137:fxp<+/-,58,25>)
                  n371 = local read "Optics Z Stage Displacement (nm)"() -> (w135:fxp<+/-,58,25>)
                  n372 = local read "X Stage External Reference (nm)"() -> (w126:fxp<+/-,58,25>)
                  n373 = local read "Y Stage External Reference (nm)"() -> (w125:fxp<+/-,58,25>)
                  n374 = local read "Z Stage External Reference (nm)"() -> (w124:fxp<+/-,58,25>)
                  n375 = local read "X Stage Reference (nm)"() -> (w146:fxp<+/-,58,25>)
                  n376 = local read "Y Stage Reference (nm)"() -> (w131:fxp<+/-,58,25>)
                  n377 = local read "Z Stage Reference (nm)"() -> (w130:fxp<+/-,58,25>)
                  n378 = local read "Detector Trigger (V)"() -> (w122:fxp<+/-,20,5>)
                  n379 = local read "PI X-Stage Input (V)"() -> (w145:fxp<+/-,20,5>)
                  n380 = local read "PI Y-Stage Input (V)"() -> (w144:fxp<+/-,20,5>)
                  n381 = local read "PI Z-Stage Input (V)"() -> (w143:fxp<+/-,20,5>)
                  n382 = case shown="\"Data Log 15\"" "Datalog Cases" {
                    tunnel: fxp<+/-,58,25> 0.0 ("fixed-point type") -> [w148 w161 w170 w183 w192 w207 w220 w232 w250 w262 w272 w284 w295 w307 w318 w330]
                    tunnel: [w157 w168 w180 w191 w204 w217 w227 w244 w254 w268 w277 w292 w304 w315 w326 w338] -> w141
                    tunnel: w146 -> [w158 _ _ _ w197 _ _ _ _ _ _ _ _ _ _ w334]
                    tunnel: w145 -> [w154 _ _ _ w196 _ _ _ _ w269 _ _ w299 _ _ _]
                    tunnel: w144 -> [_ w167 _ _ _ w211 _ _ _ _ w282 _ _ w310 _ _]
                    tunnel: w143 -> [_ _ w177 _ _ _ w224 _ _ _ _ w293 _ _ w321 _]
                    tunnel: [w156 w160 w179 w185 w203 w216 w226 w240 w253 w263 w276 w291 w303 w314 w325 w337] -> w140
                    tunnel: [w155 w169 w178 w190 w202 w215 w225 w236 w252 w264 w275 w290 w302 w313 w324 w336] -> w139
                    tunnel: w138 -> [w151 _ _ w187 w199 _ _ w247 _ w267 w281 w288 w298 _ _ w332]
                    tunnel: w137 -> [_ w163 _ w186 _ w210 _ w243 _ w266 w280 w287 _ w309 _ w331]
                    tunnel: fxp<+/-,40,17> 0.0 ("fixed-point type") -> [w150 w162 w172 w181 w194 w206 w218 w231 w248 w259 w271 w283 w297 w306 w317 _]
                    tunnel: w135 -> [_ _ w173 w184 _ _ w223 w239 _ w260 w279 w286 _ _ w320 _]
                    tunnel: w134 -> [_ _ _ _ w198 _ _ w246 w257 _ _ _ _ _ _ _]
                    tunnel: w133 -> [_ _ _ _ _ w209 _ w242 w256 _ _ _ _ _ _ _]
                    tunnel: w132 -> [_ _ _ _ _ _ w222 w238 w255 _ _ _ _ _ _ _]
                    tunnel: w131 -> [_ w166 _ _ _ w212 _ _ _ _ _ _ _ _ _ w333]
                    tunnel: w130 -> [_ _ w176 _ _ _ w228 _ _ _ _ _ _ _ _ _]
                    tunnel: [w153 w165 w175 w189 w201 w214 w221 w235 w251 w265 w274 w289 w301 w312 w323 w335] -> w129
                    tunnel: w128 -> [w152 w164 w174 w188 w200 w213 w229 w234 w258 w270 w278 w294 w305 w316 w327 w339]
                    tunnel: [w152 w164 w174 w188 w200 w213 w229 w234 w258 w270 w278 w294 w305 w316 w327 w339] -> w127
                    tunnel: w126 -> [_ _ _ _ _ _ _ _ _ _ _ _ w300 _ _ _]
                    tunnel: w125 -> [_ _ _ _ _ _ _ _ _ _ _ _ _ w311 _ _]
                    tunnel: w124 -> [_ _ _ _ _ _ _ _ _ _ _ _ _ _ w322 _]
                    tunnel: w122 -> [_ _ _ _ _ _ _ _ _ _ _ _ _ _ _ w329]
                    tunnel: [w149 w159 w171 w182 w193 w205 w219 w233 w249 w261 w273 w285 w296 w308 w319 w328] -> w121
                    frame "Data Log 1", Default {
                      n383 = To Fixed-Point(fixed-point type=w148, number=w158) -> (fixed-point=w157:fxp<+/-,58,25>)
                      n384 = To Fixed-Point(fixed-point type=w148, number=w154) -> (fixed-point=w156:fxp<+/-,58,25>)
                      n385 = To Fixed-Point(fixed-point type=w148, number=w151) -> (fixed-point=w155:fxp<+/-,58,25>)
                      n386 = To Fixed-Point(fixed-point type=w148, number=w150) -> (fixed-point=w153:fxp<+/-,58,25>)
                      n387 = To Fixed-Point(fixed-point type=w148, number=w150) -> (fixed-point=w149:fxp<+/-,58,25>)
                    }
                    frame "Data Log 2" {
                      n388 = To Fixed-Point(fixed-point type=w161, number=w166) -> (fixed-point=w168:fxp<+/-,58,25>)
                      n389 = To Fixed-Point(fixed-point type=w161, number=w167) -> (fixed-point=w160:fxp<+/-,58,25>)
                      n390 = To Fixed-Point(fixed-point type=w161, number=w163) -> (fixed-point=w169:fxp<+/-,58,25>)
                      n391 = To Fixed-Point(fixed-point type=w161, number=w162) -> (fixed-point=w165:fxp<+/-,58,25>)
                      n392 = To Fixed-Point(fixed-point type=w161, number=w162) -> (fixed-point=w159:fxp<+/-,58,25>)
                    }
                    frame "Data Log 3" {
                      n393 = To Fixed-Point(fixed-point type=w170, number=w176) -> (fixed-point=w180:fxp<+/-,58,25>)
                      n394 = To Fixed-Point(fixed-point type=w170, number=w177) -> (fixed-point=w179:fxp<+/-,58,25>)
                      n395 = To Fixed-Point(fixed-point type=w170, number=w173) -> (fixed-point=w178:fxp<+/-,58,25>)
                      n396 = To Fixed-Point(fixed-point type=w170, number=w172) -> (fixed-point=w175:fxp<+/-,58,25>)
                      n397 = To Fixed-Point(fixed-point type=w170, number=w172) -> (fixed-point=w171:fxp<+/-,58,25>)
                    }
                    frame "Data Log 4" {
                      n398 = To Fixed-Point(fixed-point type=w183, number=w187) -> (fixed-point=w191:fxp<+/-,58,25>)
                      n399 = To Fixed-Point(fixed-point type=w183, number=w186) -> (fixed-point=w185:fxp<+/-,58,25>)
                      n400 = To Fixed-Point(fixed-point type=w183, number=w184) -> (fixed-point=w190:fxp<+/-,58,25>)
                      n401 = To Fixed-Point(fixed-point type=w183, number=w181) -> (fixed-point=w189:fxp<+/-,58,25>)
                      n402 = To Fixed-Point(fixed-point type=w183, number=w181) -> (fixed-point=w182:fxp<+/-,58,25>)
                    }
                    frame "Data Log 5" {
                      n403 = To Fixed-Point(fixed-point type=w192, number=w197) -> (fixed-point=w204:fxp<+/-,58,25>)
                      n404 = Subtract(x=w199, y=w198) -> (x-y=w195:fxp<+/-,59,26>)
                      n405 = To Fixed-Point(fixed-point type=w192, number=w196) -> (fixed-point=w203:fxp<+/-,58,25>)
                      n406 = To Fixed-Point(fixed-point type=w192, number=w195) -> (fixed-point=w202:fxp<+/-,58,25>)
                      n407 = To Fixed-Point(fixed-point type=w192, number=w194) -> (fixed-point=w201:fxp<+/-,58,25>)
                      n408 = To Fixed-Point(fixed-point type=w192, number=w194) -> (fixed-point=w193:fxp<+/-,58,25>)
                    }
                    frame "Data Log 6" {
                      n409 = To Fixed-Point(fixed-point type=w207, number=w212) -> (fixed-point=w217:fxp<+/-,58,25>)
                      n410 = To Fixed-Point(fixed-point type=w207, number=w211) -> (fixed-point=w216:fxp<+/-,58,25>)
                      n411 = Subtract(x=w210, y=w209) -> (x-y=w208:fxp<+/-,59,26>)
                      n412 = To Fixed-Point(fixed-point type=w207, number=w208) -> (fixed-point=w215:fxp<+/-,58,25>)
                      n413 = To Fixed-Point(fixed-point type=w207, number=w206) -> (fixed-point=w214:fxp<+/-,58,25>)
                      n414 = To Fixed-Point(fixed-point type=w207, number=w206) -> (fixed-point=w205:fxp<+/-,58,25>)
                    }
                    frame "Data Log 7" {
                      n415 = To Fixed-Point(fixed-point type=w220, number=w228) -> (fixed-point=w227:fxp<+/-,58,25>)
                      n416 = To Fixed-Point(fixed-point type=w220, number=w224) -> (fixed-point=w226:fxp<+/-,58,25>)
                      n417 = Subtract(x=w223, y=w222) -> (x-y=w230:fxp<+/-,59,26>)
                      n418 = To Fixed-Point(fixed-point type=w220, number=w230) -> (fixed-point=w225:fxp<+/-,58,25>)
                      n419 = To Fixed-Point(fixed-point type=w220, number=w218) -> (fixed-point=w221:fxp<+/-,58,25>)
                      n420 = To Fixed-Point(fixed-point type=w220, number=w218) -> (fixed-point=w219:fxp<+/-,58,25>)
                    }
                    frame "Data Log 8" {
                      n421 = Subtract(x=w247, y=w246) -> (x-y=w245:fxp<+/-,59,26>)
                      n422 = Subtract(x=w243, y=w242) -> (x-y=w241:fxp<+/-,59,26>)
                      n423 = To Fixed-Point(fixed-point type=w232, number=w245) -> (fixed-point=w244:fxp<+/-,58,25>)
                      n424 = Subtract(x=w239, y=w238) -> (x-y=w237:fxp<+/-,59,26>)
                      n425 = To Fixed-Point(fixed-point type=w232, number=w241) -> (fixed-point=w240:fxp<+/-,58,25>)
                      n426 = To Fixed-Point(fixed-point type=w232, number=w237) -> (fixed-point=w236:fxp<+/-,58,25>)
                      n427 = To Fixed-Point(fixed-point type=w232, number=w231) -> (fixed-point=w235:fxp<+/-,58,25>)
                      n428 = To Fixed-Point(fixed-point type=w232, number=w231) -> (fixed-point=w233:fxp<+/-,58,25>)
                    }
                    frame "Data Log 9" {
                      n429 = To Fixed-Point(fixed-point type=w250, number=w257) -> (fixed-point=w254:fxp<+/-,58,25>)
                      n430 = To Fixed-Point(fixed-point type=w250, number=w256) -> (fixed-point=w253:fxp<+/-,58,25>)
                      n431 = To Fixed-Point(fixed-point type=w250, number=w255) -> (fixed-point=w252:fxp<+/-,58,25>)
                      n432 = To Fixed-Point(fixed-point type=w250, number=w248) -> (fixed-point=w251:fxp<+/-,58,25>)
                      n433 = To Fixed-Point(fixed-point type=w250, number=w248) -> (fixed-point=w249:fxp<+/-,58,25>)
                    }
                    frame "Data Log 10" {
                      n434 = To Fixed-Point(fixed-point type=w262, number=w269) -> (fixed-point=w268:fxp<+/-,58,25>)
                      n435 = To Fixed-Point(fixed-point type=w262, number=w267) -> (fixed-point=w263:fxp<+/-,58,25>)
                      n436 = To Fixed-Point(fixed-point type=w262, number=w266) -> (fixed-point=w264:fxp<+/-,58,25>)
                      n437 = To Fixed-Point(fixed-point type=w262, number=w260) -> (fixed-point=w265:fxp<+/-,58,25>)
                      n438 = To Fixed-Point(fixed-point type=w262, number=w259) -> (fixed-point=w261:fxp<+/-,58,25>)
                    }
                    frame "Data Log 11" {
                      n439 = To Fixed-Point(fixed-point type=w272, number=w282) -> (fixed-point=w277:fxp<+/-,58,25>)
                      n440 = To Fixed-Point(fixed-point type=w272, number=w281) -> (fixed-point=w276:fxp<+/-,58,25>)
                      n441 = To Fixed-Point(fixed-point type=w272, number=w280) -> (fixed-point=w275:fxp<+/-,58,25>)
                      n442 = To Fixed-Point(fixed-point type=w272, number=w279) -> (fixed-point=w274:fxp<+/-,58,25>)
                      n443 = To Fixed-Point(fixed-point type=w272, number=w271) -> (fixed-point=w273:fxp<+/-,58,25>)
                    }
                    frame "Data Log 12" {
                      n444 = To Fixed-Point(fixed-point type=w284, number=w293) -> (fixed-point=w292:fxp<+/-,58,25>)
                      n445 = To Fixed-Point(fixed-point type=w284, number=w288) -> (fixed-point=w291:fxp<+/-,58,25>)
                      n446 = To Fixed-Point(fixed-point type=w284, number=w287) -> (fixed-point=w290:fxp<+/-,58,25>)
                      n447 = To Fixed-Point(fixed-point type=w284, number=w286) -> (fixed-point=w289:fxp<+/-,58,25>)
                      n448 = To Fixed-Point(fixed-point type=w284, number=w283) -> (fixed-point=w285:fxp<+/-,58,25>)
                    }
                    frame "Data Log 13" {
                      n449 = To Fixed-Point(fixed-point type=w295, number=w300) -> (fixed-point=w304:fxp<+/-,58,25>)
                      n450 = To Fixed-Point(fixed-point type=w295, number=w299) -> (fixed-point=w303:fxp<+/-,58,25>)
                      n451 = To Fixed-Point(fixed-point type=w295, number=w298) -> (fixed-point=w302:fxp<+/-,58,25>)
                      n452 = To Fixed-Point(fixed-point type=w295, number=w297) -> (fixed-point=w301:fxp<+/-,58,25>)
                      n453 = To Fixed-Point(fixed-point type=w295, number=w297) -> (fixed-point=w296:fxp<+/-,58,25>)
                    }
                    frame "Data Log 14" {
                      n454 = To Fixed-Point(fixed-point type=w307, number=w311) -> (fixed-point=w315:fxp<+/-,58,25>)
                      n455 = To Fixed-Point(fixed-point type=w307, number=w310) -> (fixed-point=w314:fxp<+/-,58,25>)
                      n456 = To Fixed-Point(fixed-point type=w307, number=w309) -> (fixed-point=w313:fxp<+/-,58,25>)
                      n457 = To Fixed-Point(fixed-point type=w307, number=w306) -> (fixed-point=w312:fxp<+/-,58,25>)
                      n458 = To Fixed-Point(fixed-point type=w307, number=w306) -> (fixed-point=w308:fxp<+/-,58,25>)
                    }
                    frame "Data Log 15" {
                      n459 = To Fixed-Point(fixed-point type=w318, number=w322) -> (fixed-point=w326:fxp<+/-,58,25>)
                      n460 = To Fixed-Point(fixed-point type=w318, number=w321) -> (fixed-point=w325:fxp<+/-,58,25>)
                      n461 = To Fixed-Point(fixed-point type=w318, number=w320) -> (fixed-point=w324:fxp<+/-,58,25>)
                      n462 = To Fixed-Point(fixed-point type=w318, number=w317) -> (fixed-point=w323:fxp<+/-,58,25>)
                      n463 = To Fixed-Point(fixed-point type=w318, number=w317) -> (fixed-point=w319:fxp<+/-,58,25>)
                    }
                    frame "Data Log 16" {
                      n464 = To Fixed-Point(fixed-point type=w330, number=w334) -> (fixed-point=w338:fxp<+/-,58,25>)
                      n465 = To Fixed-Point(fixed-point type=w330, number=w333) -> (fixed-point=w337:fxp<+/-,58,25>)
                      n466 = To Fixed-Point(fixed-point type=w330, number=w332) -> (fixed-point=w336:fxp<+/-,58,25>)
                      n467 = To Fixed-Point(fixed-point type=w330, number=w331) -> (fixed-point=w335:fxp<+/-,58,25>)
                      n468 = To Fixed-Point(fixed-point type=w330, number=w329) -> (fixed-point=w328:fxp<+/-,58,25>)
                    }
                  }
                  "Number of Data Strings" <- w127
                  n469 = Build Array "Build Array"(w141, w140, w139, w129, w121) -> (w123:fxp<+/-,58,25>[])
                }
              }
              n470 = for {
                N: w119 -> [_]
                tunnel: w112 -> [w347] mode=indexing
                shift-right: [w345] -> w118
                shift-left: _ -> [w344]
                shift-right: [w341] -> w113
                shift-left: _ -> [w342]
                n471 = xnode "FIFO"("Element"=w347, "Timeout"="Timeout FPGA FIFO1", "error in (no error)"=w344) -> ("Timed Out?"=w343:bool, "error out"=w345:errorcluster)  [unwired: 1 in, 1 out]
                "FIFO Timed Out?" <- w343
                n472 = Or(x=w343, y=w342) -> (x .or. y?=w341:bool)
              }
              "FIFO Timed Out" <- w113
              n473 = call "measure_loop_rate_FPGA.vi"() -> ("Loop Rate (Ticks)"=→"Measured Datalog Time Period (Ticks)":u32)  [unwired: 11 in]
              n474 = local read "stop case"() -> (w114:bool)
              n475 = local read "Y scan done"() -> (w109:bool)
              n476 = local read "X scan done"() -> (w108:bool)
              n477 = Unbundle By Name "Unbundle By Name"(w118) -> ("Status?"=w117:bool)
              n478 = And(x=w109, y=w108) -> (x .and. y?=w107:bool)
              "Fly scan completed" <- w107
              n479 = Compound Arithmetic op=OR(w117, w113, w114, w107) -> (w116:bool)
              n480 = case shown="True" w116 {
                selector: w116 -> [_ w340]
                frame False {
                }
                frame True {
                  n481 = local write "stop case"(w340) -> ()
                }
              }
            }
          }
          frame "Step" {
          }
        }
        n482 = while {
          stop <- w352 stop-if-true
          n483 = local read "DT Frequency (periods/tick)"() -> (w356:fxp<+,32,0>)
          n484 = local read "DT Phase Offset (periods)"() -> (w355:fxp<+,32,0>)
          n485 = local read "DT Duty Cycle (periods)"() -> (w354:fxp<+,32,0>)
          n486 = local read "DT Reset"() -> (w353:bool)
          n487 = call "Square Wave Generator2"("frequency (periods/tick)"=w356, "reset"=w353, "phase offset (periods)"=w355, "duty cycle (periods)"=w354) -> ("square wave out"=w363:i16)  [unwired: 11 in]
          n488 = call "Loop Timer11"("Count(uSec)"="Data Trigger Time Period (uSec)") -> ()  [unwired: 1 out]
          n489 = call "measure_loop_rate_FPGA.vi"() -> ("Loop Rate (Ticks)"=→"Measured Data Trigger Time Period (Ticks)":u32)  [unwired: 11 in]
          n490 = Divide(x=w363, y=i16 32767) -> (x/y=w359:fxp<+/-,41,18>)
          n491 = To Fixed-Point(fixed-point type=fxp<+/-,58,25> 0.0, number=w359) -> (fixed-point=→"Trigger for Data":fxp<+/-,58,25>)
          n492 = local read "stop case"() -> (w352:bool)
        }
        n493 = case shown="No Error" w67 {
          selector: w67 -> [_ w104]
          tunnel: [w82 w104] -> w80
          frame No Error {
            n494 = while {
              tunnel: [w87] -> w83
              stop <- w85 stop-if-true
              w89 = fxp<+/-,58,25> 0.0 ("fixed-point type")
              n495 = xnode "FPGA I/O Node"() -> ("error out"=w87:errorcluster, "Mod3/AI0"=w100:fxp<+/-,24,5>, "Mod3/AI1"=w91:fxp<+/-,24,5>, "Mod3/AI2"=w90:fxp<+/-,24,5>)  [unwired: 4 in, 3 out]
              "Mod 3 Input AI0 (V)" <- w100
              "Mod 8 Input AI1 (V)" <- w91
              "Mod 8 Input AI2 (V)" <- w90
              n496 = call "Loop Timer6"("Count(uSec)"="Analog Input Time Period (uSec)") -> ()  [unwired: 1 out]
              n497 = Multiply(x=w90, y="Mod 3 AI2 V to nm Scaling") -> (x*y=w93:fxp<+/-,64,23>)
              n498 = Multiply(x=w91, y="Mod 3 AI1 V to nm Scaling") -> (x*y=w96:fxp<+/-,64,23>)
              n499 = Multiply(x=w100, y="Mod 3 AI0 V to nm Scaling") -> (x*y=w102:fxp<+/-,64,23>)
              n500 = To Fixed-Point(fixed-point type=w89, number=w102) -> (fixed-point=→"X Stage External Reference (nm)":fxp<+/-,58,25>)
              n501 = To Fixed-Point(fixed-point type=w89, number=w96) -> (fixed-point=→"Y Stage External Reference (nm)":fxp<+/-,58,25>)
              n502 = To Fixed-Point(fixed-point type=w89, number=w93) -> (fixed-point=→"Z Stage External Reference (nm)":fxp<+/-,58,25>)
              n503 = call "measure_loop_rate_FPGA.vi"() -> ("Loop Rate (Ticks)"=→"Measured Analog Input Time Period (Ticks)":u32)  [unwired: 11 in]
              n504 = local read "stop case"() -> (w86:bool)
              n505 = Unbundle By Name(w87) -> ("status"=w88:bool)
              n506 = Or(x=w88, y=w86) -> (x .or. y?=w85:bool)
            }
            n507 = xnode "FPGA I/O Node"("error in"=w83, "Mod3/Stop"=TRUE ("I/O Item")) -> ("error out"=w82:errorcluster)  [unwired: 1 in, 1 out]
          }
          frame Error {
          }
        }
        n508 = Merge Errors(w70, w80, w81) -> (w71:errorcluster)
        "Run Loop error" <- w71
        n509 = case shown="Error" w71 {
          tunnel: [FPGA_states."End Run" FPGA_states."Wait"] -> w72
          frame No Error {
          }
          frame Error {
            n510 = local write "stop case"(TRUE) -> ()
          }
        }
      }
      frame "End Run" {
        "End Run Error" <- w1303
      }
      frame "Shutdown" {
        n511 = xnode "FPGA I/O Node"("error in"=w1308, "System Reset"=TRUE) -> ("error out"=w1307:errorcluster)  [unwired: 1 in, 1 out]
        "Shutdown error" <- w1307
      }
    }
    "FPGA state" <- w37
  }
  n512 = node-c288(refnum<k21> "40 MHz Onboard Clock" ("Source Name"), w1) -> (w6:T14)
  n513 = while {
    stop <- FALSE stop-if-true
    w1318 = fxp<+/-,58,25> 0.0 ("fixed-point type")
    n514 = local read "32 bit Count Sample  Y"() -> (w1315:i32)
    n515 = local read "32 bit Count Sample  Z"() -> (w1312:i32)
    n516 = local read "32 bit Count Sample X"() -> (w1316:i32)
    n517 = local read "32 bit Count Optics  Y"() -> (w1332:i32)
    n518 = local read "32 bit Count Optics  Z"() -> (w1328:i32)
    n519 = local read "32 bit Count Optics X"() -> (w1338:i32)
    n520 = Multiply(x=w1338, y="Optics X Stage Resolution (nm)") -> (x*y=w1335:fxp<+/-,64,35>)
    "Optics X Stage Displacement raw (nm)" <- w1335
    n521 = Multiply(x=w1316, y="Sample X Stage Resolution (nm)") -> (x*y=w1324:fxp<+/-,64,35>)
    "Sample X Stage Displacement raw (nm)" <- w1324
    n522 = Multiply(x=w1332, y="Optics Y Stage Resolution (nm)") -> (x*y=w1330:fxp<+/-,64,35>)
    "Optics Y Stage Displacement raw (nm)" <- w1330
    n523 = Multiply(x=w1315, y="Sample Y Stage Resolution (nm)") -> (x*y=w1322:fxp<+/-,64,35>)
    "Sample Y Stage Displacement raw (nm)" <- w1322
    n524 = Multiply(x=w1328, y="Optics Z Stage Resolution (nm)") -> (x*y=w1326:fxp<+/-,64,35>)
    "Optics Z Stage Displacement raw (nm)" <- w1326
    n525 = Multiply(x=w1312, y="Sample Z Stage Resolution (nm)") -> (x*y=w1320:fxp<+/-,64,35>)
    "Sample Z Stage Displacement raw (nm)" <- w1320
    n526 = call "Loop Timer5"("Count(uSec)"="Plant Output Time Period (uSec)") -> ()  [unwired: 1 out]
    n527 = call "measure_loop_rate_FPGA.vi"() -> ("Loop Rate (Ticks)"=→"Measured Plant Output Time Period (Ticks)":u32)  [unwired: 11 in]
    n528 = To Fixed-Point(fixed-point type=w1318, number=w1335) -> (fixed-point=→"Optics X Stage Displacement (nm)":fxp<+/-,58,25>)
    n529 = To Fixed-Point(fixed-point type=w1318, number=w1330) -> (fixed-point=→"Optics Y Stage Displacement (nm)":fxp<+/-,58,25>)
    n530 = To Fixed-Point(fixed-point type=w1318, number=w1326) -> (fixed-point=→"Optics Z Stage Displacement (nm)":fxp<+/-,58,25>)
    n531 = To Fixed-Point(fixed-point type=w1318, number=w1324) -> (fixed-point=→"Sample X Stage Displacement (nm)":fxp<+/-,58,25>)
    n532 = To Fixed-Point(fixed-point type=w1318, number=w1322) -> (fixed-point=→"Sample Y Stage Displacement (nm)":fxp<+/-,58,25>)
    n533 = To Fixed-Point(fixed-point type=w1318, number=w1320) -> (fixed-point=→"Sample Z Stage Displacement (nm)":fxp<+/-,58,25>)
  }
  n534 = timed-loop {
    timing: w6 -> [_]
    timing-out: [_] -> w5
    shift-right: [w1370] -> _
    shift-left: _ -> [w1372]
    shift-right: [w1369] -> _
    shift-left: _ -> [w1371]
    shift-right: [w1391] -> _
    shift-left: w4 -> [w1388]
    shift-right: [w1390] -> _
    shift-left: u32 0 ("Tick Count(Ticks)") -> [w1389]
    shift-right: [w1361] -> _
    shift-left: _ -> [w1360]
    shift-right: [w1362] -> _
    shift-left: _ -> [w1359]
    shift-right: [w1384] -> _
    shift-left: w4 -> [w1383]
    shift-right: [w1349] -> _
    shift-left: _ -> [w1350]
    shift-right: [w1348] -> _
    shift-left: _ -> [w1351]
    shift-right: [w1378] -> _
    shift-left: w4 -> [w1377]
    shift-right: [w1367] -> _
    shift-left: _ -> [w1365]
    shift-right: [w1366] -> _
    shift-left: _ -> [w1364]
    shift-right: [w1387] -> _
    shift-left: w4 -> [w1386]
    shift-right: [w1354] -> _
    shift-left: _ -> [w1355]
    shift-right: [w1353] -> _
    shift-left: _ -> [w1356]
    shift-right: [w1381] -> _
    shift-left: w4 -> [w1380]
    shift-right: [w1344] -> _
    shift-left: _ -> [w1346]
    shift-right: [w1345] -> _
    shift-left: _ -> [w1347]
    shift-right: [w1376] -> _
    shift-left: w4 -> [w1374]
    shift-right: [w1341] -> _
    shift-left: _ -> [w1340]
    stop <- w1339 stop-if-true
    # "Tracks interferometer data"
    n535 = xnode "FPGA I/O Node"("error in"=w1340) -> ("error out"=w1363:errorcluster, "Mod4/DIO2"=w1367:bool, "Mod4/DIO3"=w1366:bool)  [unwired: 2 in, 2 out]
    "Mod4/DIO2" <- w1367
    "Mod4/DIO3" <- w1366
    n536 = xnode "FPGA I/O Node"("error in"=w1340) -> ("error out"=w1357:errorcluster, "Mod5/DIO2"=w1354:bool, "Mod5/DIO3"=w1353:bool)  [unwired: 2 in, 2 out]
    "Mod5/DIO2" <- w1354
    "Mod5/DIO3" <- w1353
    n537 = xnode "FPGA I/O Node"("error in"=w1340) -> ("error out"=w1343:errorcluster, "Mod6/DIO0"=w1349:bool, "Mod6/DIO1"=w1348:bool)  [unwired: 2 in, 2 out]
    "Mod6/DIO0" <- w1349
    "Mod6/DIO1" <- w1348
    n538 = xnode "FPGA I/O Node"("error in"=w1340) -> ("error out"=w1358:errorcluster, "Mod5/DIO0"=w1361:bool, "Mod5/DIO1"=w1362:bool)  [unwired: 2 in, 2 out]
    "Mod5/DIO0" <- w1361
    "Mod5/DIO1" <- w1362
    n539 = xnode ("FPGA I/O Node")("error in"=w1340) -> ("error out"=w1368:errorcluster, "Mod4/DIO0"=w1370:bool, "Mod4/DIO1"=w1369:bool)  [unwired: 2 in, 2 out]
    "Mod4/DIO0" <- w1370
    "Mod4/DIO1" <- w1369
    n540 = xnode "FPGA I/O Node"("error in"=w1340) -> ("error out"=w1342:errorcluster, "Mod6/DIO2"=w1344:bool, "Mod6/DIO3"=w1345:bool)  [unwired: 2 in, 2 out]
    "Mod6/DIO2" <- w1344
    "Mod6/DIO3" <- w1345
    n541 = call "Tick Count"() -> ("Tick Count(Ticks)"=w1390:u32)
    n542 = Subtract(x=w1390, y=w1389) -> (x-y=→"Measured Counter Time Period (Ticks)":u32)
    n543 = Merge Errors(w1368, w1363, w1358, w1357, w1343, w1342) -> (w1341:errorcluster)
    "Interferometer Loop Error" <- w1341
    n544 = call "Quadrature.vi"("Reset Counter"="Reset Optics X", "Quad A"=w1370, "ticks in"=w1388, "Last Quad B"=w1371, "Last Quad A"=w1372, "Quad B"=w1369) -> ("ticks out"=w1391:i32)  [unwired: 5 in]
    "32 bit Count Optics X" <- w1391
    n545 = call "Quadrature.vi"("Reset Counter"="Reset Sample X", "Quad A"=w1367, "ticks in"=w1386, "Last Quad B"=w1364, "Last Quad A"=w1365, "Quad B"=w1366) -> ("ticks out"=w1387:i32)  [unwired: 5 in]
    "32 bit Count Sample X" <- w1387
    n546 = call "Quadrature.vi"("Reset Counter"="Reset Optics Y", "Quad A"=w1361, "ticks in"=w1383, "Last Quad B"=w1359, "Last Quad A"=w1360, "Quad B"=w1362) -> ("ticks out"=w1384:i32)  [unwired: 5 in]
    "32 bit Count Optics  Y" <- w1384
    n547 = call "Quadrature.vi"("Reset Counter"="Reset Sample Y", "Quad A"=w1354, "ticks in"=w1380, "Last Quad B"=w1356, "Last Quad A"=w1355, "Quad B"=w1353) -> ("ticks out"=w1381:i32)  [unwired: 5 in]
    "32 bit Count Sample  Y" <- w1381
    n548 = call "Quadrature.vi"("Reset Counter"="Reset Optics Z", "Quad A"=w1349, "ticks in"=w1377, "Last Quad B"=w1351, "Last Quad A"=w1350, "Quad B"=w1348) -> ("ticks out"=w1378:i32)  [unwired: 5 in]
    "32 bit Count Optics  Z" <- w1378
    n549 = call "Quadrature.vi"("Reset Counter"="Reset Sample Z", "Quad A"=w1344, "ticks in"=w1374, "Last Quad B"=w1347, "Last Quad A"=w1346, "Quad B"=w1345) -> ("ticks out"=w1376:i32)  [unwired: 5 in]
    "32 bit Count Sample  Z" <- w1376
    n550 = Unbundle By Name(w1341) -> ("status"=w1339:bool)
  }
  n551 = node-c288(w5) -> ()  [unwired: 1 out]
